vi "User Calibration New_without calibration.vi"(0 "CalStatusTab":T4(tab), 1 "SetDac In Process":bool, 5 "Processed Variables":T3 {"Chamber Temperature" format="%.2f"; "Ambient Temperature" format="%.2f"; "Bath Temperature" format="%.2f"; "Det. Temperature" format="%.2f"; "Detector Chl 4" format="%.2g"; "Detector Chl 3" format="%.2g"; "Ref CO2" format="%.2g"; "Detector Chl 2" format="%.2g"; "Film Temperature" format="%.2f"; "Humidity" format="%.2f"; "Detector Chl 1" format="%.2g"}, 9 "DACSet":u16[](array[numeric]) format="%03x", 11 "time_now":timestamp format="%<%H:%M:%S>T", 12 "Coefficients_In":T2[](array[typedef]) {"Elapsed Time" format="%<%H:%M:%S>t"; "zero_utc" format="%x"; "cal_utc" format="%x"; "Pump Flow Rate" format="%0d"; "Number of Zeroes" format="%0d"; "V2C" format="%0d"; "C2V" format="%0d"; "duration" format="%<%H:%M:%S>t"; "DAC" format="%03x"; "mI" format="%.3g"; "V_(RA,15mA)" format="%0.4f"; "V_(RA,5mA)" format="%0.4f"; "Chamber Temp" format="%.1f"; "Humidity" format="%.1f"}) -> (2 "Cal Fail":bool, 3 "Calibration Complete":bool, 4 "CalStatus Out":u16, 6 "DAC Currents":sgl[](array[numeric]) caption="Currents" format="%.4g", 8 "CalGasTank":u8=5 max=7, 10 "Pump Settings":T1, 14 "Coefficients_Out":T2[](array[typedef]) {"Elapsed Time" format="%<%H:%M:%S>t"; "zero_utc" format="%x"; "cal_utc" format="%x"; "Pump Flow Rate" format="%0d"; "Number of Zeroes" format="%0d"; "V2C" format="%0d"; "C2V" format="%0d"; "duration" format="%<%H:%M:%S>t"; "DAC" format="%03x"; "mI" format="%.3g"; "V_(RA,15mA)" format="%0.4f"; "V_(RA,5mA)" format="%0.4f"; "Chamber Temp" format="%.1f"; "Humidity" format="%.1f"}, 15 "SetDac":bool)   [LabVIEW 2015]
uses:
  <vilib>/Analysis/NI_AALBase.lvlib
  <vilib>/Analysis/baseanly.llb/Mean (DBL).vi
  Controls/Calibration Coefficients.ctl
  Controls/Processed Variables.ctl
  Controls/Pump Settings.ctl
panel:
  out "I_delta 2":dbl[](array[numeric]) format="%0.4f"
  out "Error":bool
  out "Index":u16
  out "null array":i16[][](array[numeric])
  out "stage 4 - offset adjust":i16[][](array[numeric])=[[0, 3, 500, 1, 1], [1, 3, 500, 1, 1], [2, 3, 500, 1, 1], [3, 3, 500, 1, 1], [4, 3, 500, 1, 1], [5, 3, 500, 1, 1], [6, 3, 500, 1, 1], [7, 3, 500, 0, 0], [8, 3, 500, 0, 0], [9, 3, 500, 0, 0], [10, 3, 500, 0, 0], [11, 3, 500, 0, 0], [12, 3, 500, 0, 0], [13, 3, 500, 0, 0], [14, 3, 500, 0, 0], [15, 3, 500, 0, 0], [16, 3, 500, 0, 0], [17, 3, 500, 0, 0], [18, 3, 500, 0, 0], [19, 3, 500, 0, 0], [20, 3, 500, 0, 0], [21, 3, 500, 0, 0], [22, 3, 500, 0, 0], [23, 3, 500, 0, 0], [24, 3, 500, 0, 0], [25, 3, 500, 0, 0], [26, 3, 500, 0, 0], [27, 3, 500, 0, 0], [28, 3, 500, 0, 0], [29, 3, 500, 0, 0], [30, 3, 500, 0, 0], [31, 3, 500, 0, 0], [32, 3, 500, 0, 0], [33, 3, 500, 0, 0], [34, 3, 500, 0, 0], [35, 3, 500, 0, 0], [36, 3, 500, 0, 0], [37, 3, 500, 0, 0], [38, 3, 500, 0, 0], [39, 3, 500, 0, 0], [40, 3, 500, 0, 0], [41, 3, 500, 0, 0], [42, 3, 500, 0, 0], [43, 3, 500, 0, 0], [44, 3, 500, 0, 0], [45, 3, 500, 0, 0], [46, 3, 500, 0, 0], [47, 3, 500, 0, 0], [48, 3, 500, 0, 0], [49, 3, 500, 0, 0], [50, 3, 500, 0, 0], [51, 3, 500, 0, 0], [52, 3, 500, 0, 0], [53, 3, 500, 0, 0], [54, 3, 500, 0, 0], [55, 3, 500, 0, 0], [56, 3, 500, 0, 0], [57, 3, 500, 0, 0], [58, 3, 500, 0, 0], [59, 3, 500, 0, 0], [60, 3, 500, 0, 0], [61, 3, 500, 0, 0], [62, 3, 500, 0, 0], [63, 3, 500, 0, 0], [64, 3, 500, 0, 0], [65, 3, 500, 0, 0], [66, 3, 500, 0, 0], [67, 3, 500, 0, 0], [68, 3, 500, 0, 0], [69, 3, 500, 0, 0], [70, 3, 500, 0, 0], [71, 3, 500, 0, 0], [72, 3, 500, 0, 0], [73, 3, 500, 0, 0], [74, 3, 500, 0, 0], [75, 3, 500, 0, 0], [76, 3, 500, 0, 0], [77, 3, 500, 0, 0], [78, 3, 500, 0, 0], [79, 3, 500, 0, 0], [80, 3, 500, 0, 0], [81, 3, 500, 0, 0], [82, 3, 500, 0, 0], [83, 3, 500, 0, 0], [84, 3, 500, 0, 0], [85, 3, 500, 0, 0], [86, 3, 500, 0, 0], [87, 3, 500, 0, 0], [88, 3, 500, 0, 0], [89, 3, 500, 0, 0], [90, 3, 500, 0, 0], [91, 3, 500, 0, 0], [92, 3, 50, 1, 1]]
  out "stage 3 - span":i16[][](array[numeric])=[[0, 3, 500, 0, 1], [1, 3, 500, 0, 1], [2, 3, 500, 0, 1], [3, 3, 500, 0, 1], [4, 3, 500, 0, 1], [5, 3, 500, 0, 1], [6, 3, 50, 0, 1]]
  out "stage 2 - zeroing":i16[][](array[numeric])=[[0, 2, 500, 1, 0], [1, 2, 500, 1, 0], [2, 2, 500, 1, 0], [3, 2, 500, 1, 0], [4, 2, 500, 1, 0], [5, 2, 500, 1, 0], [6, 2, 50, 1, 0]]
  out "stage1 - humidity check":i16[][](array[numeric])=[[0, 1, 500, 1, 0], [1, 1, 50, 1, 0], [2, 1, 50, 1, 0], [3, 1, 50, 1, 0], [4, 1, 50, 1, 0], [5, 1, 50, 1, 0], [6, 1, 100, 0, 1], [7, 1, 150, 0, 1], [8, 1, 200, 0, 1], [9, 1, 250, 1, 0], [10, 1, 300, 1, 1], [0, 1, 350, 0, 0]]
  out "Tcal_Film":dbl format="%.2f"
  out "I_delta":dbl[](array[numeric]) format="%0.4f"
  out "Actual":u16
  in  "Lo Flow":u16=50
  out "Tcal_Det":dbl[](array[numeric]) format="%.2f"
  out "Raw_Humidity":dbl format="%.2f"
  out "Raw Chamber":dbl format="%.2f"
  in  "Quit":bool
  in  "CalFile":path
  in  "Calfiles":string[](array[string])
  out "Reference":dbl format="%.3g"
  out "Tcal_Humidity":dbl format="%.2f"
  in  "Hi Flow Setting":u16=100
  out "Progress Out":u8(slide) scale=0.0..255.0
  in  "Progress":u16(slide) scale=0.0..666.0
  out "Cal Gas":dbl=nan format="%.3g"
  in  "Skip Cal":bool
  in  "OK  7":bool
  in  "Calgas":dbl caption="Calibration Gas Concentration" format="%.2g"
  out "start time":timestamp format="%<%H:%M:%S>T"
  in  "Gas Tank":u8=5
  out "Calibration Message":enum16{"Calibration Is Required - "}(ring)
  in  "Calibration Code":T5(ring)
  out "Stable":bool
  in  "Low Humidity Threshold (%)":u16=60
  in  "Hi Humidity Threshold (%)":u16=90
  in  "Humidity Status":T6(ring)
  out "Stablizing":dbl[][](graph)
  out "Status":bool[](array[boolean])
  out "V2C":u8[](array[numeric])
  out "D'":dbl[](array[numeric]) format="%0.4f"
  out "C'":dbl[](array[numeric]) format="%0.4f"
  out "B'":dbl[](array[numeric]) format="%0.4f"
  out "A'":dbl[](array[numeric]) format="%0.4f"
  out "D":dbl[](array[numeric]) format="%0.4f"
  out "C":dbl[](array[numeric]) format="%0.4f"
  out "B":dbl[](array[numeric]) format="%0.4f"
  out "A":dbl[](array[numeric]) format="%0.4f"
  out "C2V":u8[](array[numeric])
  out "CHANNEL":string[](array[string])
  out "C0FC2V":dbl[](array[numeric]) format="%0.4f"
  out "C6FC2V":dbl[](array[numeric]) format="%0.4f"
  out "TYPE":string
  out "DATE":string
  out "CalFile Selected":path
  out "V_0d(target)":dbl[](array[numeric]) format="%0.4f"
  out "V_6d(target)":dbl[](array[numeric]) format="%0.4f"
  out "V_span(target)":dbl[](array[numeric]) format="%0.4f"
  out "BlueLED 2":bool[](array[boolean]) caption="BlueLED"
  out "DAC scale":dbl[](array[numeric]) format="%.3g"
  out "Zero":dbl[][](graph)
  out "Zero Status":T7(ring)
  out "V_RA(5mA)":dbl[](array[numeric]) format="%0.4f"
  out "V_RA(15mA)":dbl[](array[numeric]) format="%0.4f"
  out "mI":dbl[](array[numeric]) format="%.3g"
  out "delta 2":dbl=nan caption="delta" format="%.3g"
  out "CHANNEL 2":string[](array[string]) caption="CHANNEL"
  out "BlueLED":bool[](array[boolean])
  out "Zero 3":dbl[][](graph)
  out "CHANNEL 3":string[](array[string]) caption="CHANNEL"
  out "BlueLED 3":bool[](array[boolean]) caption="BlueLED"
  out "I'mBlue 2":bool[](array[boolean]) caption="BlueLED"
  out "V_RA(5mA) 2":dbl[](array[numeric]) format="%0.4f"
  out "V_RA(15mA) 2":dbl[](array[numeric]) format="%0.4f"
  out "mI 2":dbl[](array[numeric]) format="%.3g"
  out "DAC scale 2":dbl[](array[numeric]) format="%.3g"
  out "delta 3":dbl=nan caption="delta" format="%.3g"
  out "Zero Status 2":T8(ring)
  in  "OK 9":bool
  out "I_span":dbl[](array[numeric]) format="%0.4f"
  out "Step":i16[](array[numeric])
  out "DAC":u16[](array[numeric]) format="%03x"
  out "V_Span Delta":dbl[](array[numeric]) format="%0.4f"
  out "Span Good":bool[](array[boolean])
  out "I'mBlue":bool[](array[boolean]) caption="BlueLED"
  out "Span Point Calibration":dbl[][](graph)
  out "delta":dbl=nan format="%.3g"
  out "Zero Offset":dbl[][](graph)
  in  "OK 10":bool
  out "Calibration Complete -":timestamp format="%<%H:%M:%S\n%m/%d/%y>T"
  out "duration":i16 caption="mins" format="%<%H:%M:%S>t"
  out "V_0d(ImA)":dbl[](array[numeric]) format="%0.4f"
  out "V_6d(ImA)":dbl[](array[numeric]) format="%0.4f"
  out "V_0(adjust)":dbl[](array[numeric]) format="%0.4f"
  out "V_span(adjust)":dbl[](array[numeric]) format="%0.4f"
  out "Gain(adjust)":dbl[](array[numeric]) format="%0.4f"
  out "V_span(ImA)":dbl[](array[numeric]) format="%0.4f"
  out "Tcal_PCB":dbl=nan format="%.2f"
  out "Tcal_Chamber":dbl format="%.2f"
  out "elapsed time":i16 format="%<%H:%M:%S>t"
  out "Count":u8
  # "Channel 1"
  # "Channel 2"
  # "Channel 3"
  # "Channel 4"
  # "Initializing"
  # "1. Please Place Freespira On Base-Station\n \n2. Attach Cannula and Breathe Normally \n \n3. Enter Calibration Gas Concentration \n \n4. Press OK To Begin Calibration Process"
  # "Please Enter Calibration Code"
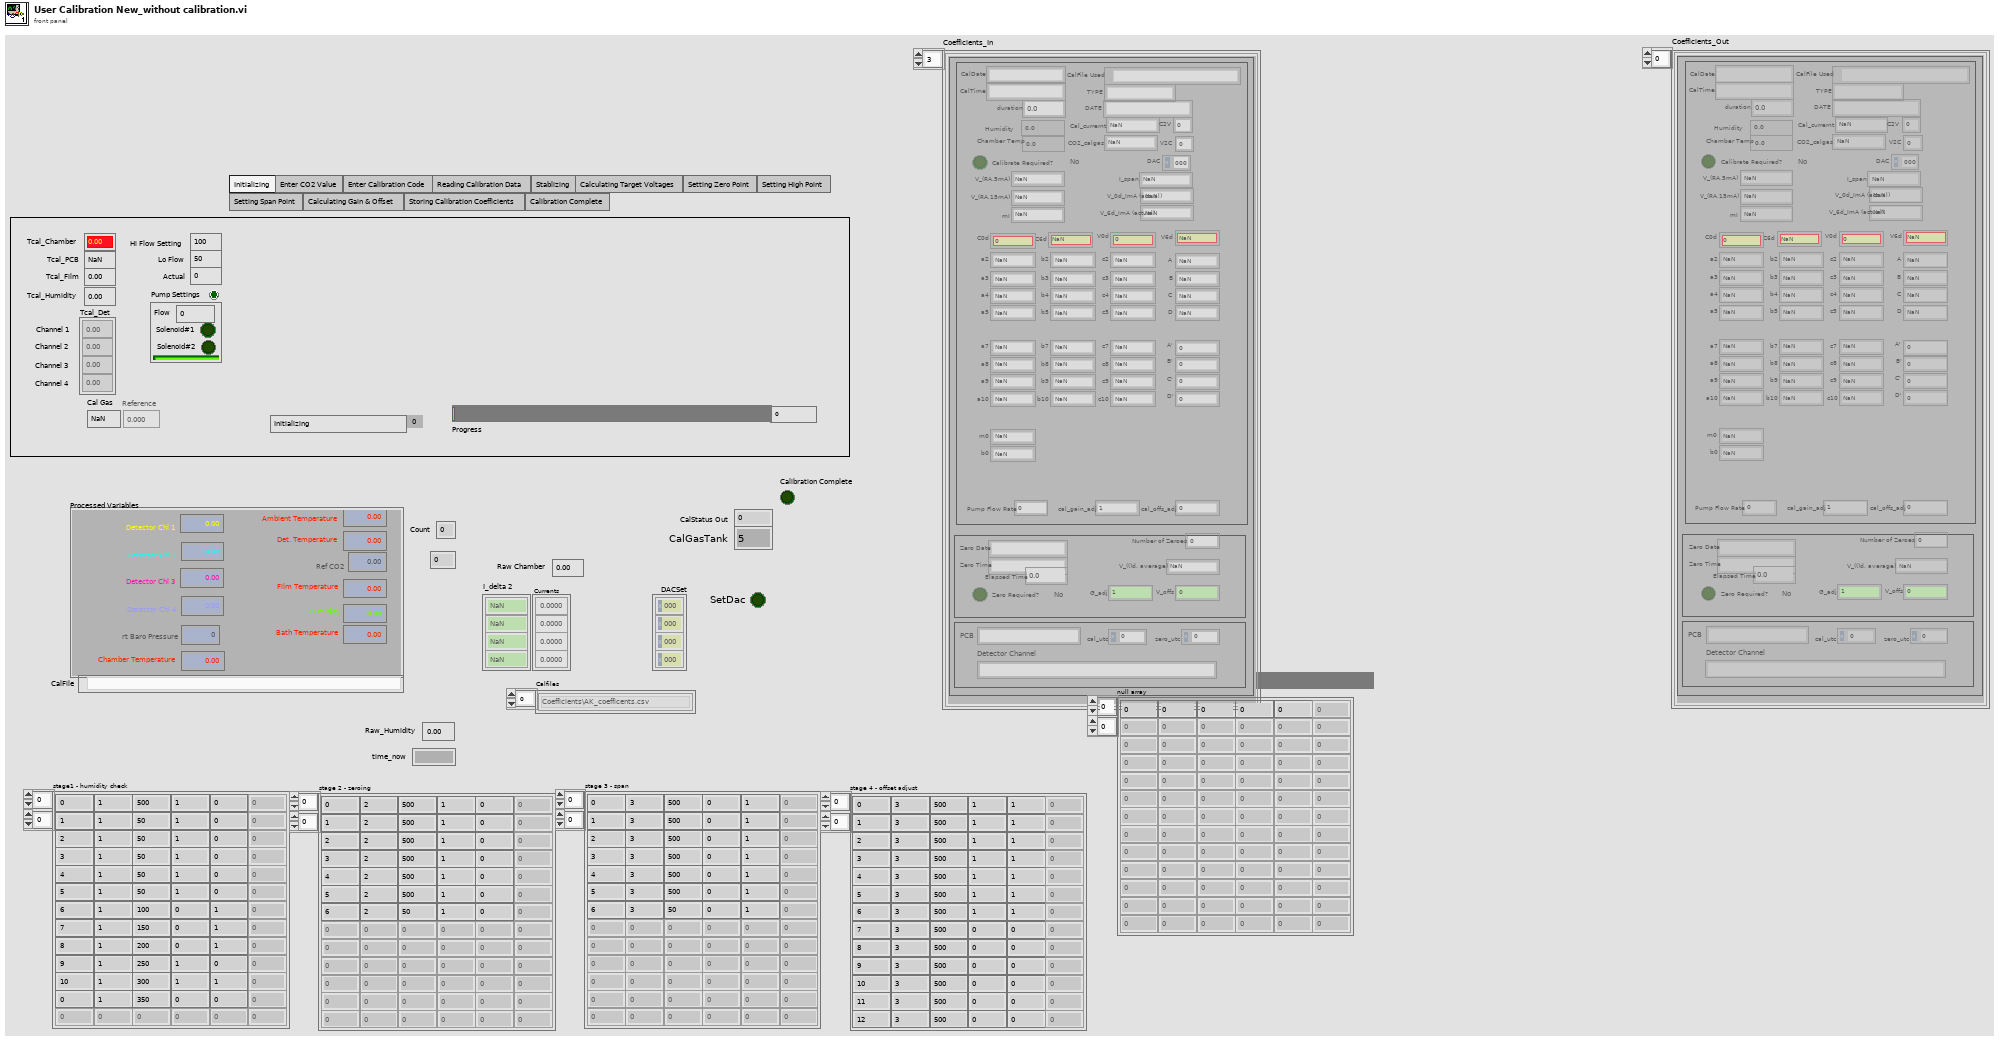
[diagram p1: front panel]
types:
  T1 = typedef "Pump Settings.ctl" = cluster{"Flow":u16, "Solenoid#1":bool, "Solenoid#2":bool, "ignore":bool}
  T2 = typedef "Calibration Coefficients.ctl" = cluster{"CalFile Used":path, "TYPE":string, "DATE":string, "Humidity":sgl, "Chamber Temp":dbl, "CO2_calgas":dbl, "V_(RA,5mA)":dbl, "V_(RA,15mA)":dbl, "mI":dbl, "V_0d_ImA (actual)":dbl, "V_6d_ImA (actual)":dbl, "I_span":dbl, "DAC":u16, "A":dbl, "B":dbl, "C":dbl, "D":dbl, "V6d":dbl, "A'":dbl, "B'":dbl, "C'":dbl, "D'":dbl, "V0d":dbl, "CalDate":string, "CalTime":string, "duration":dbl, "Detector Channel":string, "a2":dbl, "a3":dbl, "a4":dbl, "a5":dbl, "b2":dbl, "c2":dbl, "b3":dbl, "c3":dbl, "b4":dbl, "c4":dbl, "b5":dbl, "c5":dbl, "a7":dbl, "a8":dbl, "a9":dbl, "a10":dbl, "b7":dbl, "b8":dbl, "b9":dbl, "b10":dbl, "c7":dbl, "c8":dbl, "c9":dbl, "c10":dbl, "cal_offs_adj":dbl, "cal_gain_adj":dbl, "C6d":dbl, "C0d":dbl, "Cal_currernt":dbl, "C2V":u16, "V2C":u16, "Zero Date":string, "Zero Time":string, "Number of Zeroes":u16, "V_(()d, average)":dbl, "V_offs ":dbl, "G_adj":dbl, "Pump Flow Rate":u16, "Zero Required? ":bool, "Calibrate Required?":bool, "cal_utc":dbl, "zero_utc":dbl, "Elapsed Time":dbl, "PCB":string, "m0":dbl, "b0":dbl}
  T3 = typedef "Processed Variables.ctl" = cluster{"Detector Chl 1":sgl, "Humidity":dbl, "Film Temperature":dbl, "Detector Chl 2":sgl, "Ref CO2":sgl, "Detector Chl 3":sgl, "Detector Chl 4":sgl, "Det. Temperature":dbl, "Bath Temperature":dbl, "Ambient Temperature":dbl, "rt Baro Pressure":u16, "Chamber Temperature":dbl}
  T4 = enum32{"Initializing", "Enter CO2 Value", "Enter Calibration Code", "Reading Calibration Data", "Stablizing", "Calculating Target Voltages", "Setting Zero Point", "Setting High Point", "Setting Span Point", "Calculating Gain & Offset", "Storing Calibration Coefficients", "Calibration Complete"}
  T5 = enum8{"", "<User Defined>", "11111 - default", "22222 - MM_1_NS", "33333 - MM_2_S"}
  T6 = enum16{"Waiting For Film to Stabilize", "Film Stable", "Exiting", "Initializing"}
  T7 = enum16{"Setting Zero at 5 mA", "Setting Zero at 15 mA", "Calculating slopes"}
  T8 = enum16{"Setting High at 5 mA", "Setting High at 15 mA", "Calculating slopes"}
  T9 = enum32{"Invalid", "Standard", "Closed", "Hidden", "Minimized", "Maximized"}
  T10 = enum16{"Waiting For Film to Stabilize", "Film Stable - Press OK to Continue", "Exiting"}
  T11 = enum16{"Waiting For Film to Stabilize", "Film Stable - Press OK to Continue", "Exiting", "Initializing"}
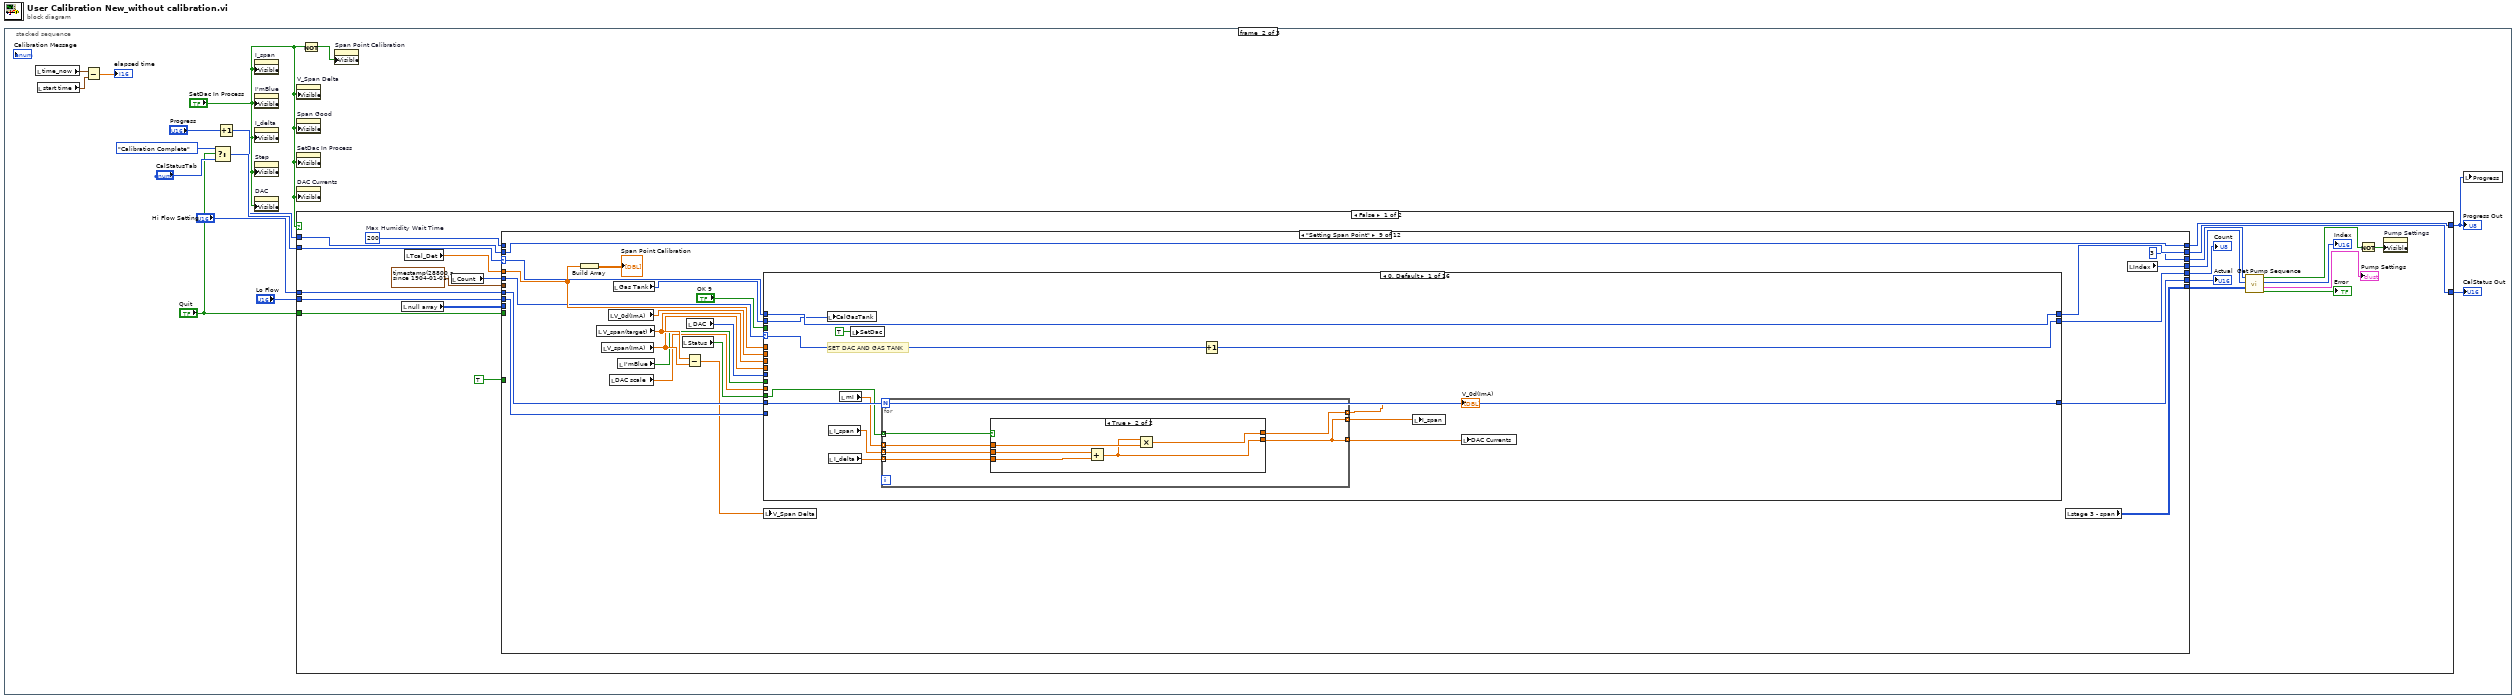
[diagram p0: block diagram]
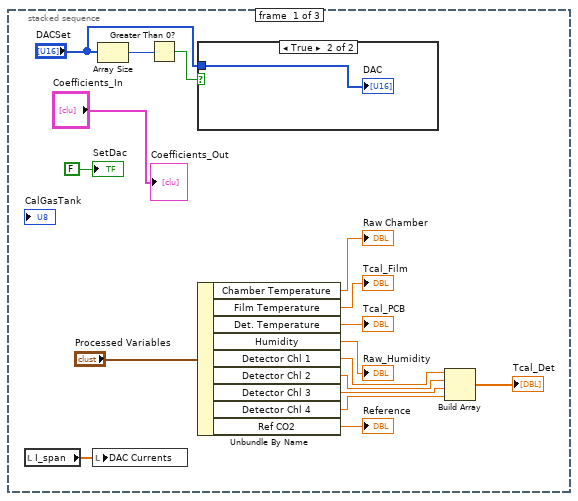
[diagram p2: hidden frame]
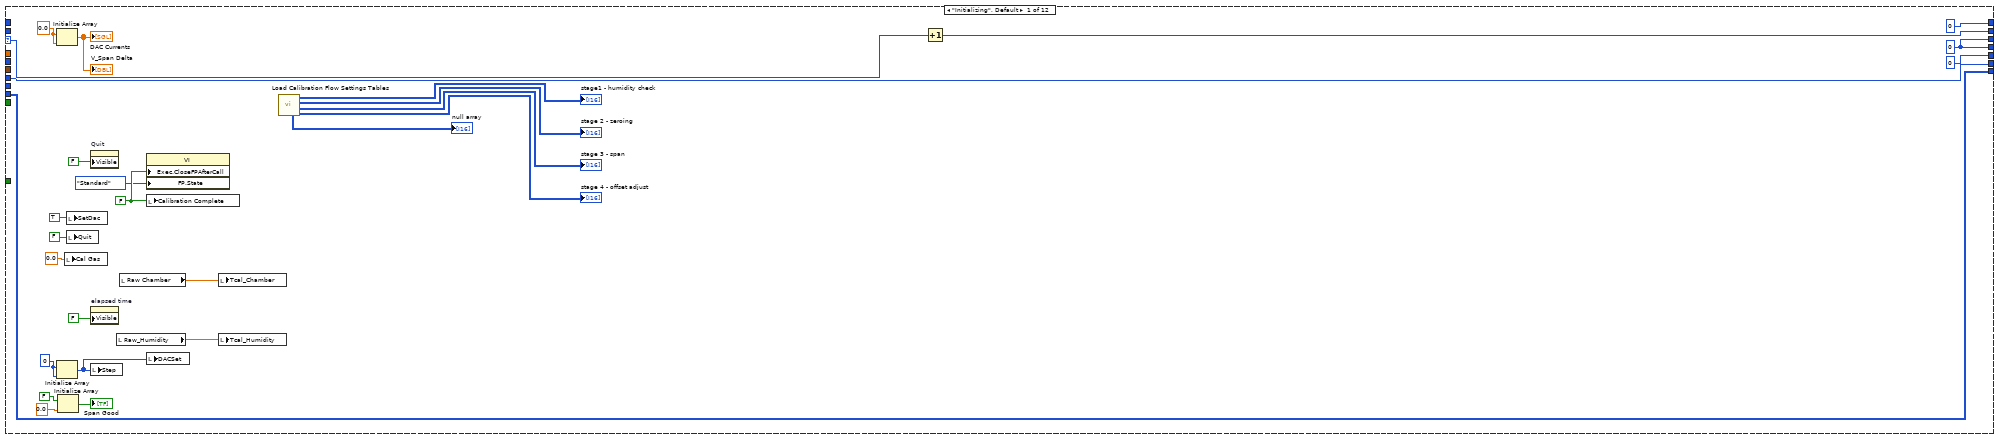
[diagram p4: hidden frame]
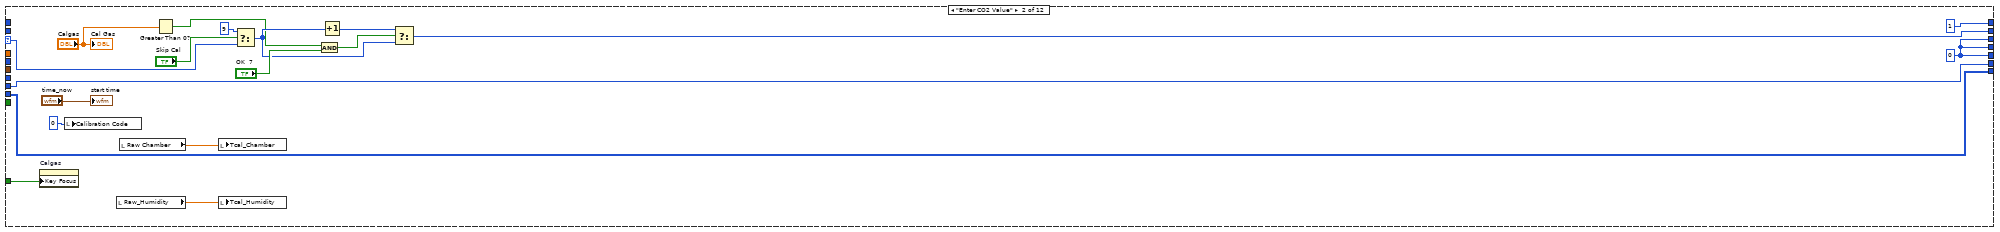
[diagram p5: hidden frame]
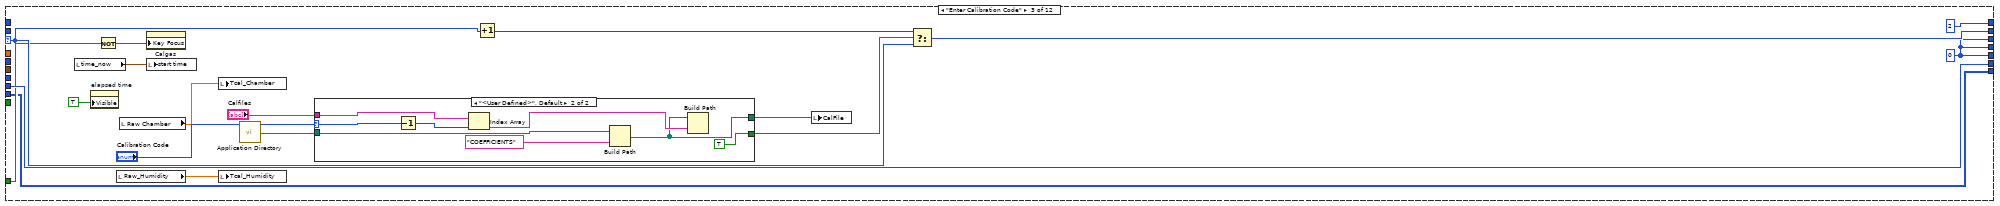
[diagram p6: hidden frame]
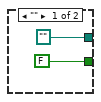
[diagram p7: hidden frame]
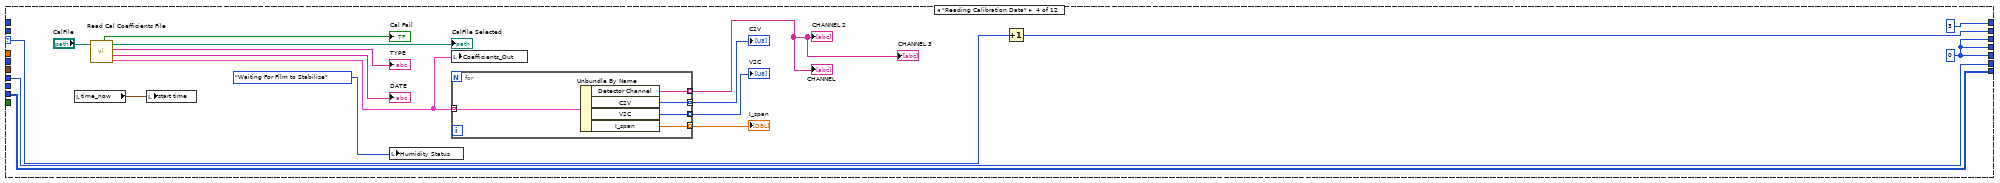
[diagram p8: hidden frame]
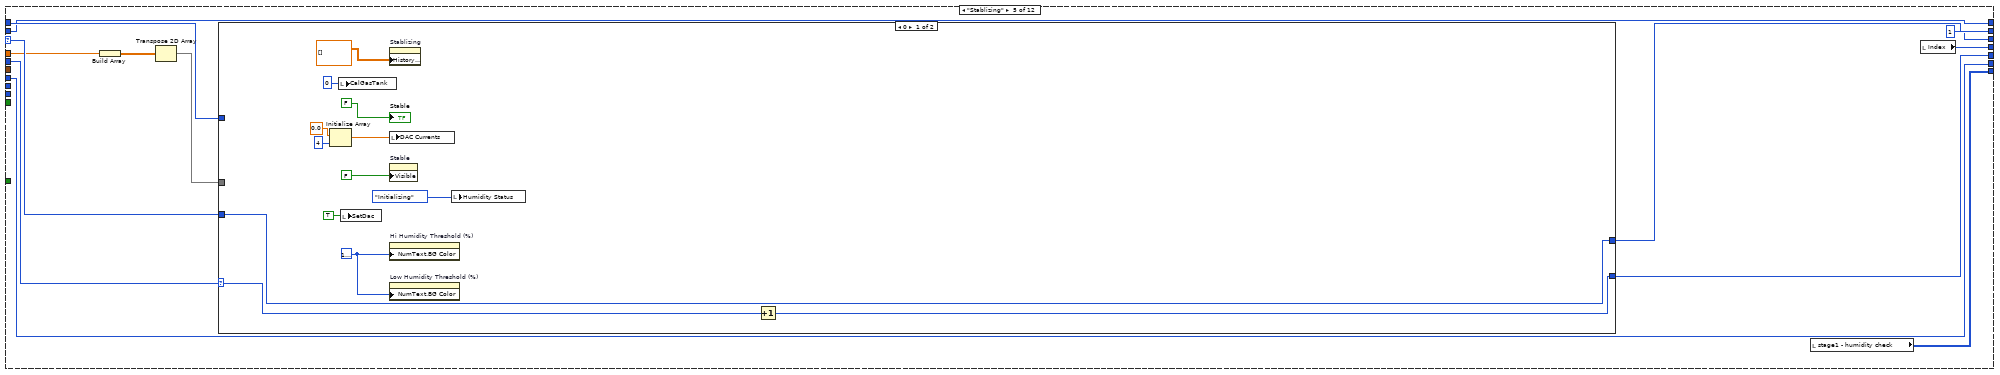
[diagram p9: hidden frame]
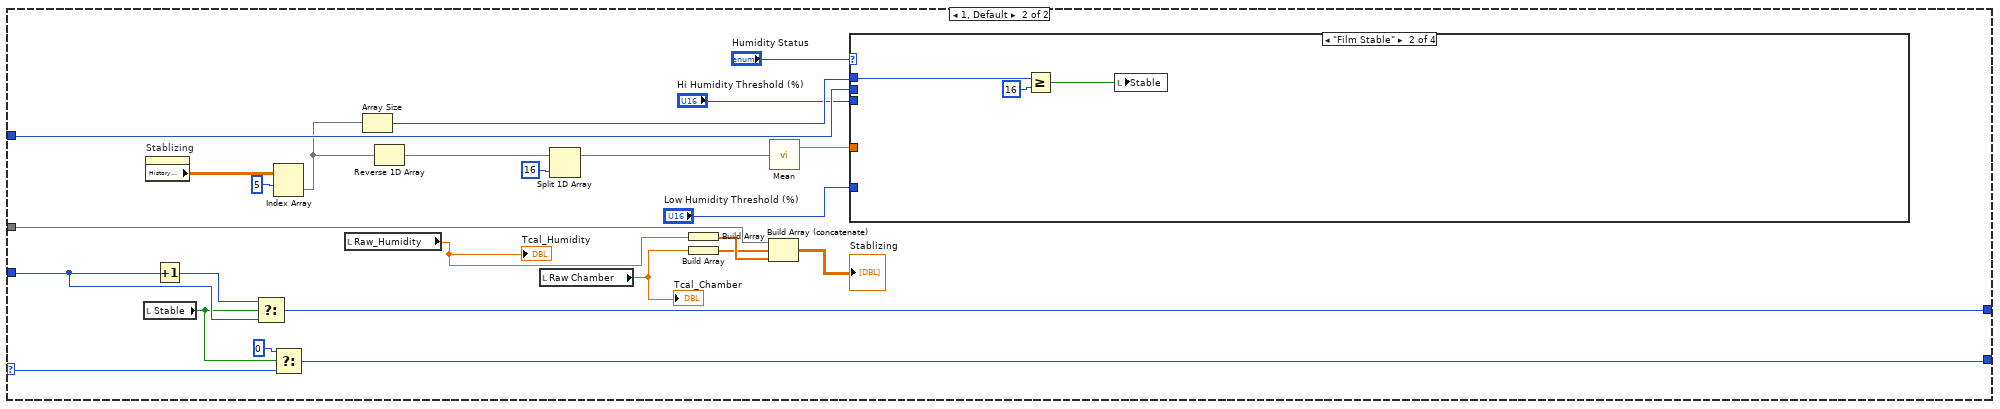
[diagram p10: hidden frame]
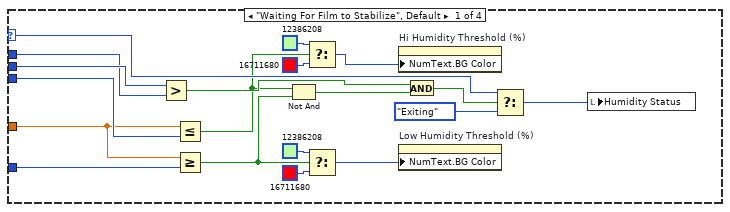
[diagram p11: hidden frame]
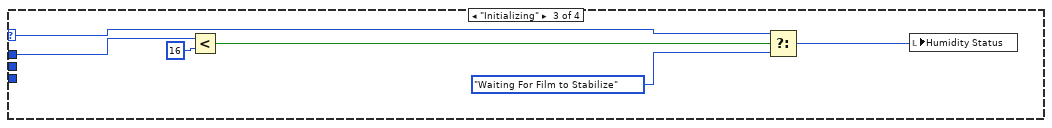
[diagram p12: hidden frame]
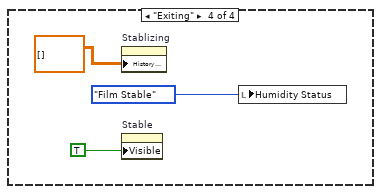
[diagram p13: hidden frame]
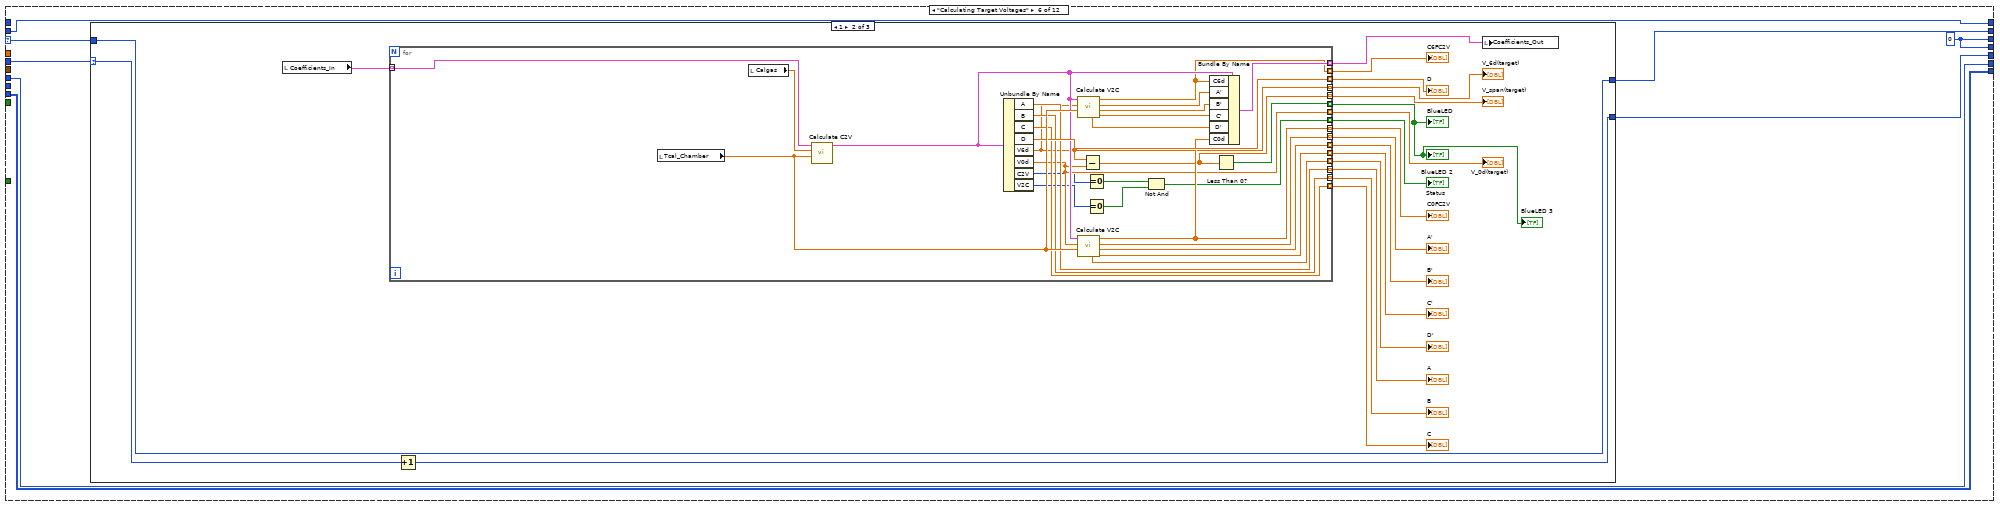
[diagram p14: hidden frame]
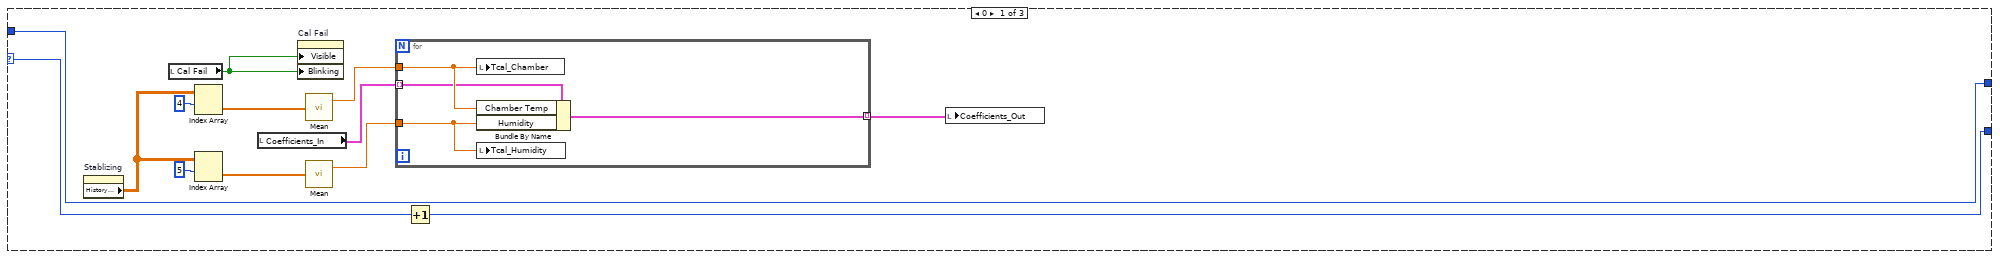
[diagram p15: hidden frame]
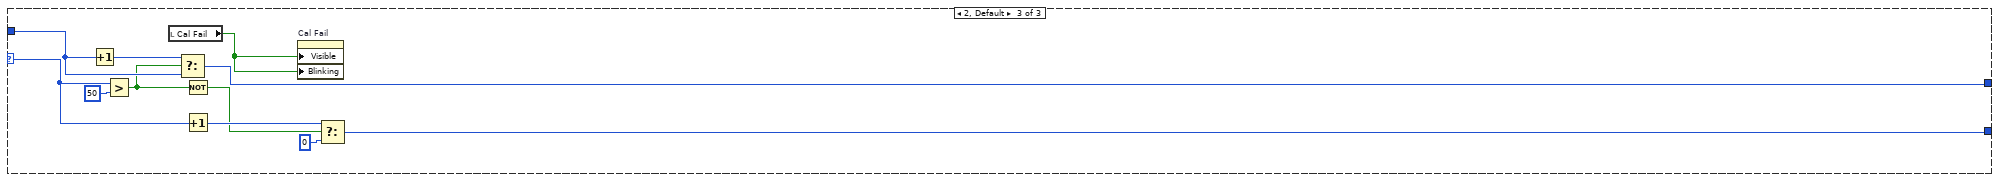
[diagram p16: hidden frame]
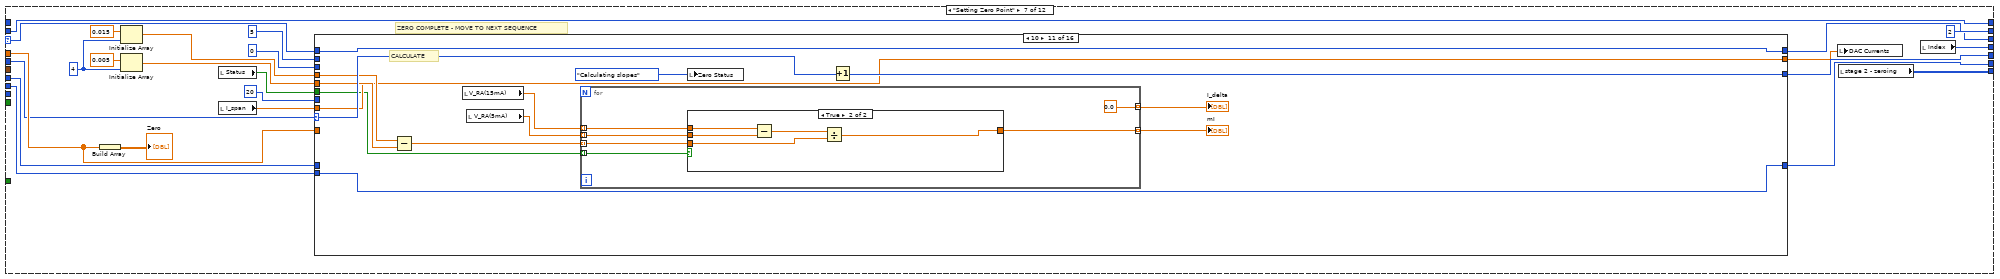
[diagram p17: hidden frame]
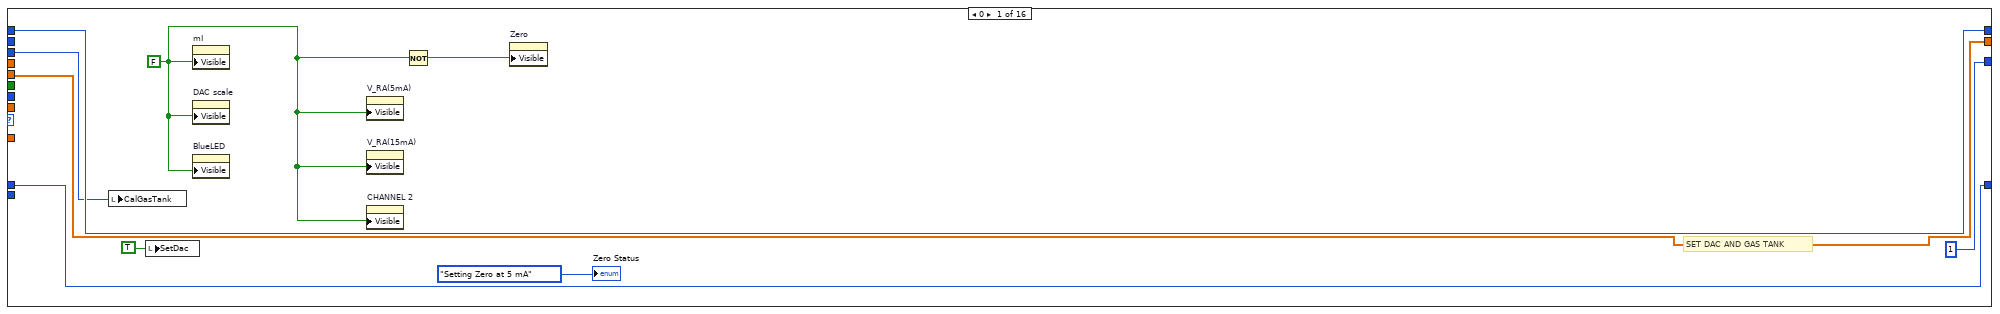
[diagram p18: hidden frame]
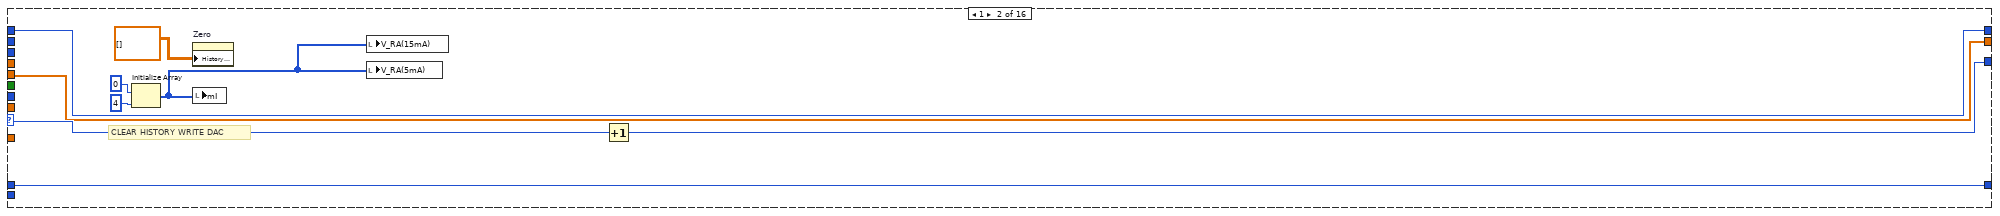
[diagram p19: hidden frame]
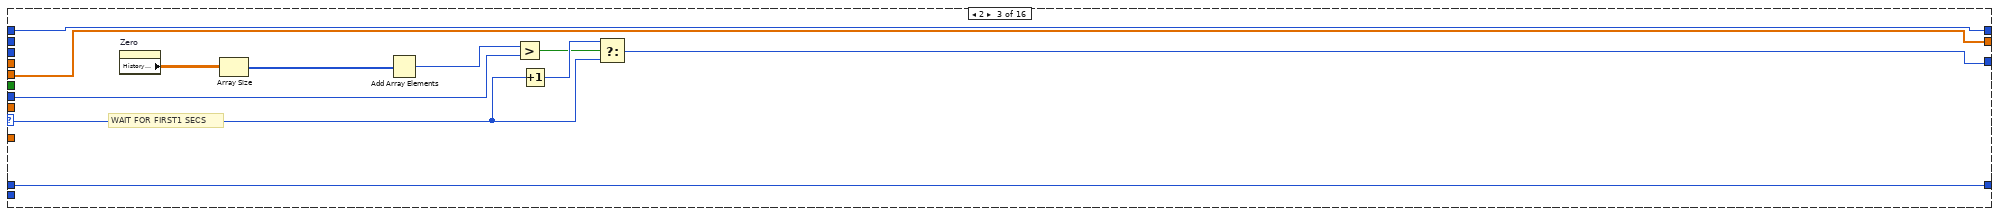
[diagram p20: hidden frame]
diagram:
  n1 = stacked-sequence {
    frame #0 {
      n2 = local read "I_span"() -> (w4:dbl[])
      n3 = local write "DAC Currents"(w4) -> ()
      n4 = Array Size(array="DACSet") -> (size(s)=w6:i32)
      n5 = Greater Than 0?(x=w6) -> (x > 0?=w5:bool)
      n6 = case shown="True" w5 {
        tunnel: "DACSet" -> [_ w18]
        frame False {
        }
        frame True {
          "DAC" <- w18
        }
      }
      n7 = Unbundle By Name("Processed Variables") -> ("Chamber Temperature"=→"Raw Chamber":dbl, "Film Temperature"=→"Tcal_Film":dbl, "Det. Temperature"=→"Tcal_PCB":dbl, "Humidity"=→"Raw_Humidity":dbl, "Detector Chl 1"=w10:sgl, "Detector Chl 2"=w9:sgl, "Detector Chl 3"=w8:sgl, "Detector Chl 4"=w12:sgl, "Ref CO2"=→"Reference":sgl)
      n8 = Build Array(w10, w9, w8, w12) -> (→"Tcal_Det":sgl[])
      "SetDac" <- FALSE
      "Coefficients_Out" <- "Coefficients_In"
    }
    frame #1 {
      n9 = local read "time_now"() -> (w29:timestamp)
      n10 = local read "start time"() -> (w30:timestamp)
      n11 = Subtract(x=w29, y=w30) -> (x-y=→"elapsed time":dbl)
      n12 = Select(t=T4."Calibration Complete" ("CalStatusTab"), s="Quit", f="CalStatusTab") -> (s? t:f=w25:T4)
      n13 = Increment(x="Progress") -> (x+1=w24:u16)
      n14 = property on="I_span" class="Arr (strict)"("Visible"="SetDac In Process") -> ()  [unwired: 2 in, 2 out]
      n15 = property on="I'mBlue" class="Arr (strict)"("Visible"="SetDac In Process") -> ()  [unwired: 2 in, 2 out]
      n16 = property on="I_delta" class="Arr (strict)"("Visible"="SetDac In Process") -> ()  [unwired: 2 in, 2 out]
      n17 = property on="Step" class="Arr (strict)"("Visible"="SetDac In Process") -> ()  [unwired: 2 in, 2 out]
      n18 = property on="DAC" class="Arr (strict)"("Visible"="SetDac In Process") -> ()  [unwired: 2 in, 2 out]
      n19 = property on="V_Span Delta" class="Arr (strict)"("Visible"="SetDac In Process") -> ()  [unwired: 2 in, 2 out]
      n20 = property on="Span Good" class="Arr (strict)"("Visible"="SetDac In Process") -> ()  [unwired: 2 in, 2 out]
      n21 = property on="SetDac In Process" class="Bool (strict)"("Visible"="SetDac In Process") -> ()  [unwired: 2 in, 2 out]
      n22 = property on="DAC Currents" class="Arr (strict)"("Visible"="SetDac In Process") -> ()  [unwired: 2 in, 2 out]
      n23 = case shown="False" "SetDac In Process" {
        tunnel: [w56 w1350] -> w33
        tunnel: [w55 w1349] -> w31
        tunnel: "Quit" -> [w51 _]
        tunnel: w25 -> [w50 w1349]
        tunnel: w24 -> [w49 w1350]
        tunnel: "Lo Flow" -> [w45 _]
        tunnel: "Hi Flow Setting" -> [w44 _]
        frame False {
          w54 = 200  # Max Humidity Wait Time
          n24 = local read "null array"() -> (w42:i16[][])
          n25 = local read "Tcal_Det"() -> (w47:dbl[])
          n26 = local read "Count"() -> (w53:u8)
          n27 = case shown="\"Setting Span Point\"" w50 {
            selector: w50 -> [w84 w93 w118 w149 w165 w244 w344 w593 w853 w1159 w1259 w1344]
            tunnel: [w80 w103 w121 w147 w164 w243 w343 w592 w852 w1158 w1258 w1344] -> w55
            tunnel: w49 -> [_ _ _ _ w163 w239 w342 w591 w851 w1160 w1257 w1343]
            tunnel: [0 1 2 3 w163 w239 w342 w591 w851 w1160 w1256 w1342] -> w56
            tunnel: w51 -> [_ _ _ _ _ _ _ _ _ _ _ _]
            tunnel: w45 -> [_ w96 w113 _ _ _ w337 w587 w848 w1153 w1255 w1340]
            tunnel: w44 -> [w77 _ _ w144 w159 w240 w336 w586 w847 w1154 _ _]
            tunnel: w54 -> [_ _ _ _ w166 _ _ _ _ _ _ _]
            tunnel: w53 -> [_ _ _ _ w158 w242 w324 w575 w835 w1147 w1254 w1341]
            tunnel: [u8 0 w85 w104 w133 w167 w241 w338 w588 w849 w1157 w1253 w1341] -> w48
            tunnel: [w77 w96 w113 w144 w159 w240 w335 w585 w846 w1156 w1252 w1340] -> w46
            tunnel: timestamp(28800 s since 1904-01-01) -> [_ _ _ _ _ _ _ _ _ _ w1251 _]
            tunnel: w47 -> [_ _ _ _ w162 _ w334 w584 w844 w1151 _ _]
            tunnel: TRUE ("Key Focus") -> [_ w87 w109 _ _ _ _ _ _ _ _ _]
            tunnel: [w58 w86 w105 w134 w157 w238 w323 w574 w834 w1148 w1250 w1338] -> w38
            tunnel: w42 -> [w58 w86 w105 w134 _ w238 _ _ _ _ w1250 w1338]
            tunnel: [w57 w85 w104 w133 1 w237 2 ("Count") 2 ("Count") 3 ("Count") 4 ("Count") w1249 w1337] -> w41
            tunnel: [w57 w85 w104 w133 w156 w237 w321 w572 w833 w1146 w1249 w1337] -> w40
            frame "Initializing", Default {
              w57 = 0
              w70 = 0.0
              w72 = 0
              w82 = FALSE ("Calibration Complete")
              n28 = Initialize Array(w70, w70) -> (→"V_Span Delta" →"DAC Currents":dbl[])
              n29 = Initialize Array(w72, w72) -> (w65:i32[])
              n30 = Initialize Array(FALSE, 0.0) -> (→"Span Good":bool[])
              n31 = local write "Cal Gas"(0.0) -> ()
              n32 = local write "SetDac"(TRUE ("SetDac")) -> ()
              n33 = local write "Quit"(FALSE ("Cal Fail")) -> ()
              n34 = property on="Quit" class="Bool (strict)"("Visible"=FALSE ("Blinking")) -> ()  [unwired: 2 in, 2 out]
              n35 = property on="elapsed time" class="DigNum (strict)"("Visible"=FALSE) -> ()  [unwired: 2 in, 2 out]
              n36 = local write "Step"(w65) -> ()
              n37 = local read "Raw_Humidity"() -> (w75:dbl)
              n38 = local read "Raw Chamber"() -> (w74:dbl)
              n39 = property class="VI"("Exec.CloseFPAfterCall"=w82, "FP.State"=T9."Standard" ("Front Panel Window:State")) -> ()  [unwired: 2 in, 2 out]
              n40 = local write "Calibration Complete"(w82) -> ()
              n41 = local write "DACSet"(w65) -> ()
              n42 = local write "Tcal_Chamber"(w74) -> ()
              n43 = local write "Tcal_Humidity"(w75) -> ()
              n44 = call "Load Calibration Flow Settings Tables.vi"() -> ("stage 4 - span"=→"stage 4 - offset adjust":i16[][], "stage 3 - high"=→"stage 3 - span":i16[][], "stage 2 - zeroing"=→"stage 2 - zeroing":i16[][], "stage1 - humidity check"=→"stage1 - humidity check":i16[][], "stage 5 - offset adjust"=→"null array":i16[][])  [unwired: 6 in, 1 out]
              n45 = Increment(x=w84) -> (x+1=w80:T4)
            }
            frame "Enter CO2 Value" {
              w85 = u8 0
              n46 = property on="Calgas" class="DigNum (strict)"("Key Focus"=w87) -> ()  [unwired: 2 in, 2 out]
              n47 = local write "Calibration Code"(0) -> ()
              n48 = local read "Raw_Humidity"() -> (w90:dbl)
              n49 = local read "Raw Chamber"() -> (w89:dbl)
              n50 = Greater Than 0?(x="Calgas") -> (x > 0?=w88:bool)
              n51 = local write "Tcal_Chamber"(w89) -> ()
              n52 = local write "Tcal_Humidity"(w90) -> ()
              n53 = Select(t=u16 9 ("CalStatus Out"), s="Skip Cal", f=w93) -> (s? t:f=w94:u32)
              n54 = And(x=w88, y="OK  7") -> (x .and. y?=w97:bool)
              n55 = Increment(x=w94) -> (x+1=w102:u32)
              n56 = Select(t=w102, s=w97, f=w94) -> (s? t:f=w103:u32)
              "start time" <- "time_now"
              "Cal Gas" <- "Calgas"
            }
            frame "Enter Calibration Code" {
              w104 = u8 0
              n57 = local read "time_now"() -> (w110:timestamp)
              n58 = property on="elapsed time" class="DigNum (strict)"("Visible"=TRUE) -> ()  [unwired: 2 in, 2 out]
              n59 = Not(x=w109) -> (.not. x?=w108:bool)
              n60 = local read "Raw_Humidity"() -> (w112:dbl)
              n61 = local read "Raw Chamber"() -> (w111:dbl)
              n62 = property on="Calgas" class="DigNum (strict)"("Key Focus"=w108) -> ()  [unwired: 2 in, 2 out]
              n63 = local write "start time"(w110) -> ()
              n64 = local write "Tcal_Chamber"(w111) -> ()
              n65 = local write "Tcal_Humidity"(w112) -> ()
              n66 = call <vilib>:"Application Directory.vi"() -> ("Application Directory"=w107:path)
              n67 = case shown="\"<User Defined>\", Default" "Calibration Code" {
                selector: "Calibration Code" -> [_ w129]
                tunnel: [FALSE TRUE] -> w117
                tunnel: "Calfiles" -> [_ w130]
                tunnel: w107 -> [_ w126]
                tunnel: [path "" w124] -> w106
                frame "" {
                }
                frame "<User Defined>", Default {
                  n68 = Decrement(x=w129) -> (x-1=w128:T5)
                  n69 = Index Array(array=w130, index=w128) -> (element=w131:string)
                  n70 = Build Path(base path=w126, name or relative path="COEFFICIENTS") -> (appended path=w124:path)
                  n71 = Build Path(base path=w124, name or relative path=w131) -> ()  [unwired: 1 out]
                }
              }
              n72 = Increment(x=w118) -> (x+1=w120:T4)
              n73 = local write "CalFile"(w106) -> ()
              n74 = Select(t=w120, s=w117, f=w118) -> (s? t:f=w121:T4)
            }
            frame "Reading Calibration Data" {
              w133 = u8 0
              n75 = local read "time_now"() -> (w145:timestamp)
              n76 = call "Read Cal Coefficients File.vi"(11:"CalFile") -> ("Original Coefficients"=w140:T2[], "DATE"=→"DATE":string, "TYPE"=→"TYPE":string, "CalFile Selected"=→"CalFile Selected":path, "Error"=→"Cal Fail":bool)  [unwired: 5 in, 1 out]
              n77 = local write "start time"(w145) -> ()
              n78 = local write "Humidity Status"(enum16{"Waiting For Film to Stabilize"}."Waiting For Film to Stabilize" ("Enum")) -> ()
              n79 = local write "Coefficients_Out"(w140) -> ()
              n80 = for {
                tunnel: w140 -> [w154] mode=indexing
                tunnel: [w153] -> w137 mode=indexing
                tunnel: [w152] -> w136 mode=indexing
                tunnel: [w151] -> w135 mode=indexing
                tunnel: [w150] -> w132 mode=indexing
                n81 = Unbundle By Name(w154) -> ("Detector Channel"=w150:string, "C2V"=w151:u16, "V2C"=w152:u16, "I_span"=w153:dbl)
              }
              "I_span" <- w137
              "V2C" <- w136
              "C2V" <- w135
              "CHANNEL" <- w132
              "CHANNEL 2" <- w132
              "CHANNEL 3" <- w132
              n82 = Increment(x=w149) -> (x+1=w147:T4)
            }
            frame "Stablizing" {
              n83 = Build Array(w162) -> (w161:dbl[][])
              n84 = Transpose 2D Array(2D array=w161) -> (transposed array=w160:dbl[][])
              n85 = case shown="0" w158 {
                selector: w158 -> [w180 w200]
                tunnel: [w179 w201] -> w167
                tunnel: w166 -> [_ w195]
                tunnel: w165 -> [w178 w199]
                tunnel: [w178 w198] -> w164
                tunnel: w160 -> [_ w182]
                frame 0 {
                  w172 = u32 16777216
                  n86 = Initialize Array(0.0, 4 ("dimension size")) -> (w170:dbl[])
                  n87 = local write "CalGasTank"(u8 0 ("CalGasTank")) -> ()
                  n88 = local write "SetDac"(TRUE ("InCal")) -> ()
                  n89 = property on="Stablizing" class="WFChart (strict)"("History Data"=dbl[][] []) -> ()  [unwired: 2 in, 2 out]
                  n90 = local write "DAC Currents"(w170) -> ()
                  n91 = property on="Stable" class="Bool (strict)"("Visible"=FALSE) -> ()  [unwired: 2 in, 2 out]
                  n92 = property on="Hi Humidity Threshold (%)" class="DigNum (strict)"("NumText.BG Color"=w172) -> ()  [unwired: 2 in, 2 out]
                  n93 = property on="Low Humidity Threshold (%)" class="DigNum (strict)"("NumText.BG Color"=w172) -> ()  [unwired: 2 in, 2 out]
                  n94 = local write "Humidity Status"(T6."Initializing" ("Humidity Status")) -> ()
                  n95 = Increment(x=w180) -> (x+1=w179:u8)
                  "Stable" <- FALSE ("Done")
                }
                frame 1, Default {
                  n96 = local read "Stable"() -> (w181:bool)
                  n97 = property on="Stablizing" class="WFChart (strict)"() -> ("History Data"=w203:dbl[][])  [unwired: 2 in, 2 out]
                  n98 = Increment(x=w199) -> (x+1=w202:T4)
                  n99 = Select(t=w202, s=w181, f=w199) -> (s? t:f=w198:T4)
                  n100 = Index Array(array=w203, index (row)=5) -> (element=w190:dbl[])  [unwired: 1 in]
                  n101 = Select(t=u8 0, s=w181, f=w200) -> (s? t:f=w201:u8)
                  n102 = local read "Raw_Humidity"() -> (w184:dbl)
                  "Tcal_Humidity" <- w184
                  n103 = Array Size(array=w190) -> (size(s)=w197:i32)
                  n104 = Reverse 1D Array(array=w190) -> (reversed array=w191:dbl[])
                  n105 = local read "Raw Chamber"() -> (w183:dbl)
                  "Tcal_Chamber" <- w183
                  n106 = Split 1D Array(array=w191, index=16) -> (first subarray=w192:dbl[])  [unwired: 1 out]
                  n107 = Build Array(w184) -> (w187:dbl[])
                  n108 = Build Array(w183) -> (w185:dbl[])
                  n109 = Build Array (concatenate)(w182, w185, w187) -> (→"Stablizing":dbl[][])
                  n110 = call-poly <vilib>:"Mean.vi"("X"=w192) -> ("mean"=w189:dbl)  [unwired: 1 out]
                  n111 = case shown="\"Film Stable\"" "Humidity Status" {
                    selector: "Humidity Status" -> [w221 _ w228 _]
                    tunnel: w197 -> [w215 w227 w233 _]
                    tunnel: w195 -> [w216 _ _ _]
                    tunnel: "Hi Humidity Threshold (%)" -> [w223 _ _ _]
                    tunnel: "Low Humidity Threshold (%)" -> [w222 _ _ _]
                    tunnel: w189 -> [w217 _ _ _]
                    frame "Waiting For Film to Stabilize", Default {
                      n112 = Greater?(x=w216, y=w215) -> (0:w220:bool)
                      n113 = Less Or Equal?(x=w217, y=w223) -> (x <= y?=w210:bool)
                      n114 = Greater Or Equal?(x=w217, y=w222) -> (x >= y?=w212:bool)
                      n115 = Not And(1:w212, 2:w210) -> (0:w218:bool)
                      n116 = Select(t=u32 12386208, s=w210, f=u32 16711680) -> (s? t:f=w211:u32)
                      n117 = Select(t=u32 12386208, s=w212, f=u32 16711680) -> (s? t:f=w213:u32)
                      n118 = property on="Hi Humidity Threshold (%)" class="DigNum (strict)"("NumText.BG Color"=w211) -> ()  [unwired: 2 in, 2 out]
                      n119 = property on="Low Humidity Threshold (%)" class="DigNum (strict)"("NumText.BG Color"=w213) -> ()  [unwired: 2 in, 2 out]
                      n120 = And(x=w220, y=w218) -> (x .and. y?=w219:bool)
                      n121 = Select(t=w221, s=w219, f=T10."Exiting" ("Humidity Status")) -> (s? t:f=w224:u16)
                      n122 = local write "Humidity Status"(w224) -> ()
                    }
                    frame "Film Stable" {
                      n123 = Greater Or Equal?(x=w227, y=16) -> (x >= y?=w225:bool)
                      n124 = local write "Stable"(w225) -> ()
                    }
                    frame "Initializing" {
                      n125 = Less?(x=w233, y=16) -> (x < y?=w231:bool)
                      n126 = Select(t=w228, s=w231, f=T11."Waiting For Film to Stabilize" ("Humidity Status")) -> (s? t:f=w230:u16)
                      n127 = local write "Humidity Status"(w230) -> ()
                    }
                    frame "Exiting" {
                      n128 = property on="Stablizing" class="WFChart (strict)"("History Data"=dbl[][] []) -> ()  [unwired: 2 in, 2 out]
                      n129 = property on="Stable" class="Bool (strict)"("Visible"=TRUE) -> ()  [unwired: 2 in, 2 out]
                      n130 = local write "Humidity Status"(T6."Film Stable" ("Humidity Status")) -> ()
                    }
                  }
                }
              }
              n131 = local read "stage1 - humidity check"() -> (w157:i16[][])
              n132 = local read "Index"() -> (w156:u16)
            }
            frame "Calculating Target Voltages" {
              w237 = u8 0 ("Count")
              n133 = case shown="1" w242 {
                selector: w242 -> [w249 w281 w320]
                tunnel: w244 -> [w250 w264 w318]
                tunnel: [w250 w264 w317] -> w243
                tunnel: [w248 w278 w312] -> w241
                frame 0 {
                  n134 = property on="Stablizing" class="WFChart (strict)"() -> ("History Data"=w253:dbl[][])  [unwired: 2 in, 2 out]
                  n135 = local read "Cal Fail"() -> (w245:bool)
                  n136 = Index Array(array=w253, index (row)=4) -> (element=w256:dbl[])  [unwired: 1 in]
                  n137 = Index Array(array=w253, index (row)=5) -> (element=w255:dbl[])  [unwired: 1 in]
                  n138 = local read "Coefficients_In"() -> (w247:T2[])
                  n139 = property on="Cal Fail" class="Bool (strict)"("Visible"=w245, "Blinking"=w245) -> ()  [unwired: 2 in, 2 out]
                  n140 = call-poly <vilib>:"Mean.vi"("X"=w256) -> ("mean"=w252:dbl)  [unwired: 1 out]
                  n141 = call-poly <vilib>:"Mean.vi"("X"=w255) -> ("mean"=w251:dbl)  [unwired: 1 out]
                  n142 = for {
                    tunnel: w252 -> [w261]
                    tunnel: [w260] -> w246 mode=indexing
                    tunnel: w251 -> [w259]
                    tunnel: w247 -> [w258] mode=indexing
                    n143 = local write "Tcal_Chamber"(w261) -> ()
                    n144 = Bundle By Name(cluster=w258, "Chamber Temp"=w261, "Humidity"=w259) -> (w260:T2)
                    n145 = local write "Tcal_Humidity"(w259) -> ()
                  }
                  n146 = Increment(x=w249) -> (x+1=w248:u8)
                  n147 = local write "Coefficients_Out"(w246) -> ()
                }
                frame 1 {
                  n148 = local read "Coefficients_In"() -> (w280:T2[])
                  n149 = for {
                    tunnel: w280 -> [w307] mode=indexing
                    tunnel: [w306] -> w279 mode=indexing
                    tunnel: [w283] -> w277 mode=indexing
                    tunnel: [w290] -> w266 mode=indexing
                    tunnel: [w305] -> w276 mode=indexing
                    tunnel: [w304] -> w275 mode=indexing
                    tunnel: [w303] -> w274 mode=indexing
                    tunnel: [w298] -> w273 mode=indexing
                    tunnel: [w302] -> w269 mode=indexing
                    tunnel: [w301] -> w270 mode=indexing
                    tunnel: [w300] -> w271 mode=indexing
                    tunnel: [w299] -> w272 mode=indexing
                    tunnel: [w297] -> w268 mode=indexing
                    tunnel: [w291] -> w267 mode=indexing
                    tunnel: [w289] -> w265 mode=indexing
                    tunnel: [w284] -> w263 mode=indexing
                    tunnel: [w282] -> w262 mode=indexing
                    n150 = local read "Tcal_Chamber"() -> (w309:dbl)
                    n151 = local read "Calgas"() -> (w308:dbl)
                    n152 = call "Calculate C2V.vi"("Tcal_Chamber"=w309, "CO2"=w308, "Calibration Coefficients"=w307) -> ("Calibration Coefficients Out"=w292:T2)  [unwired: 8 in]
                    n153 = Unbundle By Name(w292) -> ("A"=w298:dbl, "B"=w303:dbl, "C"=w304:dbl, "D"=w305:dbl, "V6d"=w290:dbl, "V0d"=w289:dbl, "C2V"=w287:u16, "V2C"=w288:u16)
                    n154 = call "Calculate V2C.vi"("Tcal_Chamber"=w309, "Voltage In"=w290, "Calibration Coefficients"=w292) -> ("C'"=w294:dbl, "B'"=w295:dbl, "A'"=w296:dbl, "CO2 Out"=w291:dbl, "D'"=w293:dbl)  [unwired: 4 in]
                    n155 = call "Calculate V2C.vi"("Tcal_Chamber"=w309, "Voltage In"=w289, "Calibration Coefficients"=w292) -> ("C'"=w300:dbl, "B'"=w301:dbl, "A'"=w302:dbl, "CO2 Out"=w297:dbl, "D'"=w299:dbl)  [unwired: 4 in]
                    n156 = Subtract(x=w290, y=w289) -> (x-y=w283:dbl)
                    n157 = Equal To 0?(x=w287) -> (x = 0?=w285:bool)
                    n158 = Equal To 0?(x=w288) -> (x = 0?=w286:bool)
                    n159 = Not And(1:w286, 2:w285) -> (0:w284:bool)
                    n160 = Bundle By Name(cluster=w292, "C6d"=w291, "A'"=w296, "B'"=w295, "C'"=w294, "D'"=w293, "C0d"=w297) -> (w306:T2)
                    n161 = Less Than 0?(x=w283) -> (x < 0?=w282:bool)
                  }
                  "V_0d(target)" <- w265
                  "V_6d(target)" <- w266
                  "V_span(target)" <- w277
                  "C6FC2V" <- w267
                  "A" <- w273
                  "B" <- w274
                  "C" <- w275
                  "D" <- w276
                  "B'" <- w270
                  "C'" <- w271
                  "D'" <- w272
                  "A'" <- w269
                  "C0FC2V" <- w268
                  "Status" <- w263
                  "BlueLED" <- w262
                  "BlueLED 2" <- w262
                  "BlueLED 3" <- w262
                  n162 = Increment(x=w281) -> (x+1=w278:u8)
                  n163 = local write "Coefficients_Out"(w279) -> ()
                }
                frame 2, Default {
                  n164 = Increment(x=w318) -> (x+1=w316:T4)
                  n165 = Greater?(x=w320, y=u8 50) -> (0:w313:bool)
                  n166 = local read "Cal Fail"() -> (w310:bool)
                  n167 = Select(t=w316, s=w313, f=w318) -> (s? t:f=w317:T4)
                  n168 = Not(x=w313) -> (.not. x?=w311:bool)
                  n169 = Increment(x=w320) -> (x+1=w315:u8)
                  n170 = property on="Cal Fail" class="Bool (strict)"("Visible"=w310, "Blinking"=w310) -> ()  [unwired: 2 in, 2 out]
                  n171 = Select(t=w315, s=w311, f=u8 0) -> (s? t:f=w312:u8)
                }
              }
            }
            frame "Setting Zero Point" {
              w330 = 4 ("index")
              # "ZERO COMPLETE - MOVE TO NEXT SEQUENCE"
              n172 = Build Array(w334) -> (→"Zero":dbl[][])
              n173 = Initialize Array(0.015, w330) -> (w329:dbl[])
              n174 = Initialize Array(0.005, w330) -> (w328:dbl[])
              n175 = local read "Status"() -> (w325:bool[])
              n176 = local read "I_span"() -> (w326:dbl[])
              n177 = case shown="10" w324 {
                selector: w324 -> [_ w362 w373 w378 w399 w428 w434 w445 w450 w466 w503 w523 w533 w557 w562 _]
                tunnel: [1 w361 w371 w376 w398 w427 w433 w443 w448 w465 w504 w522 w532 w556 w561 0] -> w338
                tunnel: w344 -> [w353 w360 w370 w377 w400 w426 w432 w442 w449 w473 w506 w524 w531 w558 w563 w568]
                tunnel: [w353 w360 w370 w377 w400 w426 w432 w442 w449 w473 w506 w524 w531 w558 w563 w567] -> w343
                tunnel: 20 ("y") -> [_ _ w367 _ _ _ _ w439 _ _ _ _ _ _ _ _]
                tunnel: w337 -> [_ _ _ w375 w394 w422 w430 w436 w447 w472 w505 w525 w535 w552 w564 w566]
                tunnel: w336 -> [w349 w358 w366 _ _ _ _ _ _ _ _ _ _ _ _ _]
                tunnel: 5 ("index") -> [_ _ _ _ _ _ _ _ _ _ _ _ _ _ _ _]
                tunnel: u8 0 ("CalGasTank") -> [w351 _ _ _ _ w424 _ _ _ _ _ _ _ _ _ _]
                tunnel: w328 -> [w346 w354 w363 w374 w388 _ _ _ _ _ w501 _ _ _ _ _]
                tunnel: w329 -> [_ _ _ _ _ w421 w429 w435 w446 w460 w502 _ _ _ _ _]
                tunnel: [w349 w358 w366 w375 w394 w422 w430 w436 w447 w472 w505 w525 w535 w552 w564 w566] -> w335
                tunnel: w334 -> [_ _ _ _ w392 _ _ _ _ w464 _ _ _ _ _ _]
                tunnel: [w346 w354 w363 w374 w388 w421 w429 w435 w446 w460 w494 w520 w530 w559 w560 w565] -> w327
                tunnel: w326 -> [_ _ _ _ _ _ _ _ _ _ w494 w520 w530 w559 w560 w565]
                tunnel: w325 -> [_ _ _ _ w379 _ _ _ _ w451 w493 _ _ _ _ _]
                frame 0 {
                  w345 = FALSE ("Visible")
                  # "SET DAC AND GAS TANK"
                  n178 = local write "CalGasTank"(w351) -> ()
                  n179 = local write "SetDac"(TRUE ("InCal")) -> ()
                  n180 = property on="mI" class="Arr (strict)"("Visible"=w345) -> ()  [unwired: 2 in, 2 out]
                  n181 = property on="DAC scale" class="Arr (strict)"("Visible"=w345) -> ()  [unwired: 2 in, 2 out]
                  n182 = property on="BlueLED" class="Arr (strict)"("Visible"=w345) -> ()  [unwired: 2 in, 2 out]
                  n183 = property on="V_RA(5mA)" class="Arr (strict)"("Visible"=w345) -> ()  [unwired: 2 in, 2 out]
                  n184 = property on="V_RA(15mA)" class="Arr (strict)"("Visible"=w345) -> ()  [unwired: 2 in, 2 out]
                  n185 = property on="CHANNEL 2" class="Arr (strict)"("Visible"=w345) -> ()  [unwired: 2 in, 2 out]
                  n186 = Not(x=w345) -> (.not. x?=w347:bool)
                  n187 = property on="Zero" class="WFChart (strict)"("Visible"=w347) -> ()  [unwired: 2 in, 2 out]
                  "Zero Status" <- T7."Setting Zero at 5 mA" ("Zero Status")
                }
                frame 1 {
                  # "CLEAR HISTORY WRITE DAC"
                  n188 = Initialize Array(0, 4 ("dimension size")) -> (w356:i32[])
                  n189 = property on="Zero" class="WFChart (strict)"("History Data"=dbl[][] []) -> ()  [unwired: 2 in, 2 out]
                  n190 = local write "mI"(w356) -> ()
                  n191 = local write "V_RA(15mA)"(w356) -> ()
                  n192 = local write "V_RA(5mA)"(w356) -> ()
                  n193 = Increment(x=w362) -> (x+1=w361:u8)
                }
                frame 2 {
                  # "WAIT FOR FIRST1 SECS"
                  n194 = property on="Zero" class="WFChart (strict)"() -> ("History Data"=w368:dbl[][])  [unwired: 2 in, 2 out]
                  n195 = Array Size(array=w368) -> (size(s)=w365:i32[])
                  n196 = Add Array Elements(numeric array=w365) -> (sum=w364:i32)
                  n197 = Greater?(x=w364, y=w367) -> (0:w369:bool)
                  n198 = Increment(x=w373) -> (x+1=w372:u8)
                  n199 = Select(t=w372, s=w369, f=w373) -> (s? t:f=w371:u8)
                }
                frame 3 {
                  # "IGNORE FIRST1 SECS - RESET AIRFLOW"
                  n200 = Increment(x=w378) -> (x+1=w376:u8)
                }
                frame 4 {
                  # "RUN TEST UNTIL STABLE"
                  n201 = property on="Zero" class="WFChart (strict)"() -> ("History Data"=w390:dbl[][])  [unwired: 2 in, 2 out]
                  n202 = Transpose 2D Array(2D array=w390) -> (transposed array=w389:dbl[][])
                  n203 = for {
                    tunnel: w389 -> [w407] mode=indexing
                    tunnel: w392 -> [w406] mode=indexing
                    tunnel: [w405] -> w387 mode=indexing
                    tunnel: [w404] -> w391 mode=indexing
                    tunnel: [w403] -> w380 mode=indexing
                    tunnel: w379 -> [w402] mode=indexing
                    n204 = case shown="True" w402 {
                      tunnel: w407 -> [_ w415]
                      tunnel: w406 -> [_ w414]
                      tunnel: [TRUE w413] -> w405
                      tunnel: [0.0 ("mean") w412] -> w404
                      tunnel: [0.0 w411] -> w403
                      frame False {
                      }
                      frame True {
                        n205 = Reverse 1D Array(array=w415) -> (reversed array=w416:dbl[])
                        n206 = Split 1D Array(array=w416, index=16) -> (first subarray=w417:dbl[])  [unwired: 1 out]
                        n207 = call-poly <vilib>:"Mean.vi"("X"=w417) -> ("mean"=w412:dbl)  [unwired: 1 out]
                        n208 = Subtract(x=w412, y=w414) -> (x-y=w419:dbl)
                        n209 = Absolute Value(x=w419) -> (abs(x)=w411:dbl)
                        n210 = Less Or Equal?(x=w411, y=0.001) -> (x <= y?=w413:bool)
                      }
                    }
                  }
                  "V_RA(5mA)" <- w391
                  n211 = Array Size(array=w389) -> (size(s)=w397:i32[])
                  n212 = Add Array Elements(numeric array=w397) -> (sum=w382:i32)
                  n213 = Greater?(x=w382, y=40 ("index")) -> (0:w395:bool)
                  n214 = Increment(x=w399) -> (x+1=w401:u8)
                  n215 = Greater?(x=w382, y=100 ("index")) -> (0:w383:bool)
                  n216 = Add Array Elements(numeric array=w380) -> (sum=w381:dbl)
                  n217 = And Array Elements(Boolean array=w387) -> (logical AND=w386:bool)
                  n218 = local write "delta 2"(w381) -> ()
                  n219 = And(x=w395, y=w386) -> (x .and. y?=w384:bool)
                  n220 = Compound Arithmetic op=OR(w383, w384) -> (w393:bool)
                  n221 = Select(t=w401, s=w393, f=w399) -> (s? t:f=w398:u8)
                }
                frame 5 {
                  # "SET DAC AND GAS TANK"
                  n222 = local write "CalGasTank"(w424) -> ()
                  n223 = local write "SetDac"(TRUE ("InCal")) -> ()
                  n224 = local write "Zero Status"(T7."Setting Zero at 15 mA" ("Zero Status")) -> ()
                  n225 = Increment(x=w428) -> (x+1=w427:u8)
                }
                frame 6 {
                  # "CLEAR HISTORY WRITE DAC"
                  n226 = property on="Zero" class="WFChart (strict)"("History Data"=dbl[][] []) -> ()  [unwired: 2 in, 2 out]
                  n227 = Increment(x=w434) -> (x+1=w433:u8)
                }
                frame 7 {
                  # "WAIT FOR FIRST 1 SECS"
                  n228 = property on="Zero" class="WFChart (strict)"() -> ("History Data"=w440:dbl[][])  [unwired: 2 in, 2 out]
                  n229 = Array Size(array=w440) -> (size(s)=w441:i32[])
                  n230 = Add Array Elements(numeric array=w441) -> (sum=w438:i32)
                  n231 = Greater?(x=w438, y=w439) -> (0:w437:bool)
                  n232 = Increment(x=w445) -> (x+1=w444:u8)
                  n233 = Select(t=w444, s=w437, f=w445) -> (s? t:f=w443:u8)
                }
                frame 8 {
                  # "IGNORE FIRST 1 SECS - RESET AIRFLOW"
                  n234 = Increment(x=w450) -> (x+1=w448:u8)
                }
                frame 9 {
                  # "RUN TEST UNTIL STABLE"
                  n235 = property on="Zero" class="WFChart (strict)"() -> ("History Data"=w462:dbl[][])  [unwired: 2 in, 2 out]
                  n236 = Transpose 2D Array(2D array=w462) -> (transposed array=w461:dbl[][])
                  n237 = for {
                    tunnel: w461 -> [w479] mode=indexing
                    tunnel: w464 -> [w478] mode=indexing
                    tunnel: [w477] -> w459 mode=indexing
                    tunnel: [w476] -> w463 mode=indexing
                    tunnel: [w475] -> w452 mode=indexing
                    tunnel: w451 -> [w474] mode=indexing
                    n238 = case shown="True" w474 {
                      tunnel: w479 -> [_ w487]
                      tunnel: w478 -> [_ w486]
                      tunnel: [TRUE w485] -> w477
                      tunnel: [0.0 ("mean") w484] -> w476
                      tunnel: [0.0 w483] -> w475
                      frame False {
                      }
                      frame True {
                        n239 = Reverse 1D Array(array=w487) -> (reversed array=w488:dbl[])
                        n240 = Split 1D Array(array=w488, index=16) -> (first subarray=w489:dbl[])  [unwired: 1 out]
                        n241 = call-poly <vilib>:"Mean.vi"("X"=w489) -> ("mean"=w484:dbl)  [unwired: 1 out]
                        n242 = Subtract(x=w484, y=w486) -> (x-y=w491:dbl)
                        n243 = Absolute Value(x=w491) -> (abs(x)=w483:dbl)
                        n244 = Less Or Equal?(x=w483, y=0.001) -> (x <= y?=w485:bool)
                      }
                    }
                  }
                  "V_RA(15mA)" <- w463
                  n245 = Array Size(array=w461) -> (size(s)=w470:i32[])
                  n246 = Add Array Elements(numeric array=w470) -> (sum=w455:i32)
                  n247 = Greater?(x=w455, y=40 ("index")) -> (0:w468:bool)
                  n248 = Increment(x=w466) -> (x+1=w471:u8)
                  n249 = Greater?(x=w455, y=100 ("index")) -> (0:w454:bool)
                  n250 = Add Array Elements(numeric array=w452) -> (sum=→"delta 2":dbl)
                  n251 = And Array Elements(Boolean array=w459) -> (logical AND=w458:bool)
                  n252 = And(x=w468, y=w458) -> (x .and. y?=w457:bool)
                  n253 = Compound Arithmetic op=OR(w454, w457) -> (w467:bool)
                  n254 = Select(t=w471, s=w467, f=w466) -> (s? t:f=w465:u8)
                }
                frame 10 {
                  # "CALCULATE"
                  n255 = Subtract(x=w502, y=w501) -> (x-y=w500:dbl[])
                  n256 = local read "V_RA(15mA)"() -> (w498:dbl[])
                  n257 = local read "V_RA(5mA)"() -> (w499:dbl[])
                  n258 = for {
                    tunnel: w500 -> [w510] mode=indexing
                    tunnel: w499 -> [w511] mode=indexing
                    tunnel: w498 -> [w512] mode=indexing
                    tunnel: [w509] -> w497 mode=indexing
                    tunnel: [0.0 ("x*y")] -> w495 mode=indexing
                    tunnel: w493 -> [w507] mode=indexing
                    n259 = case shown="True" w507 {
                      tunnel: w512 -> [_ w518]
                      tunnel: w511 -> [_ w517]
                      tunnel: w510 -> [_ w515]
                      tunnel: [0.0 w514] -> w509
                      frame False {
                      }
                      frame True {
                        n260 = Subtract(x=w518, y=w517) -> (x-y=w516:dbl)
                        n261 = Divide(x=w516, y=w515) -> (x/y=w514:dbl)
                      }
                    }
                  }
                  "mI" <- w497
                  "I_delta" <- w495
                  n262 = local write "Zero Status"(T7."Calculating slopes" ("Zero Status")) -> ()
                  n263 = Increment(x=w503) -> (x+1=w504:u8)
                }
                frame 11 {
                  w519 = TRUE ("Visible")
                  # "ZERO COMPLETE - Display and wait one sec"
                  n264 = property on="mI" class="Arr (strict)"("Visible"=w519) -> ()  [unwired: 2 in, 2 out]
                  n265 = property on="BlueLED" class="Arr (strict)"("Visible"=w519) -> ()  [unwired: 2 in, 2 out]
                  n266 = property on="DAC scale" class="Arr (strict)"("Visible"=w519) -> ()  [unwired: 2 in, 2 out]
                  n267 = property on="V_RA(5mA)" class="Arr (strict)"("Visible"=w519) -> ()  [unwired: 2 in, 2 out]
                  n268 = property on="V_RA(15mA)" class="Arr (strict)"("Visible"=w519) -> ()  [unwired: 2 in, 2 out]
                  n269 = property on="CHANNEL 2" class="Arr (strict)"("Visible"=w519) -> ()  [unwired: 2 in, 2 out]
                  n270 = Not(x=w519) -> (.not. x?=w521:bool)
                  n271 = property on="Zero" class="WFChart (strict)"("Visible"=w521) -> ()  [unwired: 2 in, 2 out]
                  n272 = Increment(x=w523) -> (x+1=w522:u8)
                }
                frame 12 {
                  n273 = local write "OK 9"(FALSE) -> ()
                  n274 = local read "Coefficients_In"() -> (w539:T2[])
                  n275 = local read "V_RA(15mA)"() -> (w536:dbl[])
                  n276 = local read "V_RA(5mA)"() -> (w537:dbl[])
                  n277 = local read "BlueLED"() -> (w526:bool[])
                  n278 = local read "mI"() -> (w540:dbl[])
                  n279 = for {
                    tunnel: w540 -> [w544] mode=indexing
                    tunnel: w539 -> [w551] mode=indexing
                    tunnel: [w550] -> w538 mode=indexing
                    tunnel: w537 -> [w549] mode=indexing
                    tunnel: w536 -> [w548] mode=indexing
                    tunnel: [0.0] -> w529 mode=indexing
                    tunnel: [i8 0 ("Step")] -> w534 mode=indexing
                    tunnel: [w543] -> w528 mode=indexing
                    tunnel: [w542] -> w527 mode=indexing
                    tunnel: w526 -> [w542] mode=indexing
                    n280 = Bundle By Name(cluster=w551, "V_(RA,5mA)"=w549, "V_(RA,15mA)"=w548, "mI"=w544) -> (w550:T2)
                    n281 = Divide(x=50, y=w544) -> (x/y=w543:dbl)
                  }
                  "DAC scale" <- w528
                  "I'mBlue" <- w527
                  n282 = Increment(x=w533) -> (x+1=w532:u8)
                  n283 = local write "Step"(w534) -> ()
                  n284 = local write "I_delta"(w529) -> ()
                  n285 = local write "Coefficients_Out"(w538) -> ()
                }
                frame 13 {
                  # "Set DAC to start calgas early"
                  n286 = local read "I_span"() -> (w554:dbl[])
                  n287 = local write "SetDac"(TRUE ("InCal")) -> ()
                  n288 = local write "DAC Currents"(w554) -> ()
                  n289 = local read "Gas Tank"() -> (w555:u8)
                  n290 = local write "CalGasTank"(w555) -> ()
                  n291 = Increment(x=w557) -> (x+1=w556:u8)
                }
                frame 14, Default {
                  # "ZERO COMPLETE - Display and wait one sec"
                  n292 = Increment(x=w562) -> (x+1=w561:u8)
                }
                frame 30 {
                  n293 = Increment(x=w568) -> (x+1=w567:T4)
                }
              }
              n294 = local write "DAC Currents"(w327) -> ()
              n295 = local read "stage 2 - zeroing"() -> (w323:i16[][])
              n296 = local read "Index"() -> (w321:u16)
            }
            frame "Setting High Point" {
              w581 = 4 ("index")
              # "ZERO COMPLETE - MOVE TO NEXT SEQUENCE"
              n297 = Build Array(w584) -> (→"Zero 3":dbl[][])
              n298 = Initialize Array(0.005, w581) -> (w579:dbl[])
              n299 = Initialize Array(0.015, w581) -> (w580:dbl[])
              n300 = local read "Status"() -> (w576:bool[])
              n301 = local read "I_span"() -> (w577:dbl[])
              n302 = case shown="13" w575 {
                selector: w575 -> [_ w605 w623 w634 w639 w660 w689 w695 w706 w711 w727 w764 w784 w794 w818 w823 _]
                tunnel: [1 w606 w622 w632 w637 w659 w688 w694 w704 w709 w726 w765 w783 w793 w817 w822 0] -> w588
                tunnel: w593 -> [w603 w604 w621 w631 w638 w661 w687 w693 w703 w710 w734 w767 w785 w792 w819 w824 w829]
                tunnel: [w603 w604 w621 w631 w638 w661 w687 w693 w703 w710 w734 w767 w785 w792 w819 w824 w828] -> w592
                tunnel: 20 ("y") -> [_ _ _ w628 _ _ _ _ w700 _ _ _ _ _ _ _ _]
                tunnel: w587 -> [_ _ _ _ w636 w655 w683 w691 w697 w708 w733 w766 w786 w796 w813 w825 w827]
                tunnel: w586 -> [w599 w613 w619 w627 _ _ _ _ _ _ _ _ _ _ _ _ _]
                tunnel: 5 ("index") -> [_ _ _ _ _ _ _ _ _ _ _ _ _ _ _ _ _]
                tunnel: "Gas Tank" -> [w601 _ _ _ _ _ w685 _ _ _ _ _ _ _ _ _ _]
                tunnel: w579 -> [w596 _ w615 w624 w635 w649 _ _ _ _ _ w762 _ _ _ _ _]
                tunnel: w580 -> [_ _ _ _ _ _ w682 w690 w696 w707 w721 w763 _ _ _ _ _]
                tunnel: [w599 w613 w619 w627 w636 w655 w683 w691 w697 w708 w733 w766 w786 w796 w813 w825 w827] -> w585
                tunnel: w584 -> [_ _ _ _ _ w653 _ _ _ _ w725 _ _ _ _ _ _]
                tunnel: [w596 w614 w615 w624 w635 w649 w682 w690 w696 w707 w721 w755 w781 w791 w820 w821 w826] -> w578
                tunnel: w577 -> [_ w614 _ _ _ _ _ _ _ _ _ w755 w781 w791 w820 w821 w826]
                tunnel: w576 -> [_ _ _ _ _ w640 _ _ _ _ w712 w754 _ _ _ _ _]
                frame 0 {
                  w595 = FALSE ("Visible")
                  # "SET DAC AND GAS TANK"
                  # "SET DAC AND GAS TANK"
                  n303 = local write "CalGasTank"(w601) -> ()
                  n304 = local write "SetDac"(TRUE ("InCal")) -> ()
                  n305 = property on="mI 2" class="Arr (strict)"("Visible"=w595) -> ()  [unwired: 2 in, 2 out]
                  n306 = property on="BlueLED" class="Arr (strict)"("Visible"=w595) -> ()  [unwired: 2 in, 2 out]
                  n307 = property on="Zero 3" class="WFChart (strict)"("History Data"=dbl[][] []) -> ()  [unwired: 2 in, 2 out]
                  n308 = property on="V_RA(5mA) 2" class="Arr (strict)"("Visible"=w595) -> ()  [unwired: 2 in, 2 out]
                  n309 = property on="V_RA(15mA) 2" class="Arr (strict)"("Visible"=w595) -> ()  [unwired: 2 in, 2 out]
                  n310 = property on="DAC scale 2" class="Arr (strict)"("Visible"=w595) -> ()  [unwired: 2 in, 2 out]
                  n311 = property on="CHANNEL 3" class="Arr (strict)"("Visible"=w595) -> ()  [unwired: 2 in, 2 out]
                  n312 = Not(x=w595) -> (.not. x?=w597:bool)
                  n313 = property on="Zero 3" class="WFChart (strict)"("Visible"=w597) -> ()  [unwired: 2 in, 2 out]
                  "Zero Status 2" <- T8."Setting High at 5 mA" ("Zero Status 2")
                }
                frame 1 {
                  n314 = property on="Zero 3" class="WFChart (strict)"() -> ("History Data"=w612:dbl[][])  [unwired: 2 in, 2 out]
                  n315 = Array Size(array=w612) -> (size(s)=w611:i32[])
                  n316 = Increment(x=w605) -> (x+1=w609:u8)
                  n317 = Add Array Elements(numeric array=w611) -> (sum=w607:i32)
                  n318 = Greater?(x=w607, y=10) -> (0:w608:bool)
                  n319 = Select(t=w609, s=w608, f=w605) -> (s? t:f=w606:u8)
                }
                frame 2 {
                  # "CLEAR HISTORY WRITE DAC"
                  n320 = Initialize Array(0, 4 ("dimension size")) -> (w617:i32[])
                  n321 = property on="Zero 3" class="WFChart (strict)"("History Data"=dbl[][] []) -> ()  [unwired: 2 in, 2 out]
                  n322 = local write "mI 2"(w617) -> ()
                  n323 = local write "V_RA(15mA) 2"(w617) -> ()
                  n324 = local write "V_RA(5mA) 2"(w617) -> ()
                  n325 = Increment(x=w623) -> (x+1=w622:u8)
                }
                frame 3 {
                  # "WAIT FOR FIRST1 SECS"
                  n326 = property on="Zero 3" class="WFChart (strict)"() -> ("History Data"=w629:dbl[][])  [unwired: 2 in, 2 out]
                  n327 = Array Size(array=w629) -> (size(s)=w626:i32[])
                  n328 = Add Array Elements(numeric array=w626) -> (sum=w625:i32)
                  n329 = Greater?(x=w625, y=w628) -> (0:w630:bool)
                  n330 = Increment(x=w634) -> (x+1=w633:u8)
                  n331 = Select(t=w633, s=w630, f=w634) -> (s? t:f=w632:u8)
                }
                frame 4 {
                  # "IGNORE FIRST1 SECS - RESET AIRFLOW"
                  n332 = Increment(x=w639) -> (x+1=w637:u8)
                }
                frame 5 {
                  # "RUN TEST UNTIL STABLE"
                  n333 = property on="Zero 3" class="WFChart (strict)"() -> ("History Data"=w651:dbl[][])  [unwired: 2 in, 2 out]
                  n334 = Transpose 2D Array(2D array=w651) -> (transposed array=w650:dbl[][])
                  n335 = for {
                    tunnel: w650 -> [w668] mode=indexing
                    tunnel: w653 -> [w667] mode=indexing
                    tunnel: [w666] -> w648 mode=indexing
                    tunnel: [w665] -> w652 mode=indexing
                    tunnel: [w664] -> w641 mode=indexing
                    tunnel: w640 -> [w663] mode=indexing
                    n336 = case shown="True" w663 {
                      tunnel: w668 -> [_ w676]
                      tunnel: w667 -> [_ w675]
                      tunnel: [TRUE w674] -> w666
                      tunnel: [0.0 ("mean") w673] -> w665
                      tunnel: [0.0 w672] -> w664
                      frame False {
                      }
                      frame True {
                        n337 = Reverse 1D Array(array=w676) -> (reversed array=w677:dbl[])
                        n338 = Split 1D Array(array=w677, index=16) -> (first subarray=w678:dbl[])  [unwired: 1 out]
                        n339 = call-poly <vilib>:"Mean.vi"("X"=w678) -> ("mean"=w673:dbl)  [unwired: 1 out]
                        n340 = Subtract(x=w673, y=w675) -> (x-y=w680:dbl)
                        n341 = Absolute Value(x=w680) -> (abs(x)=w672:dbl)
                        n342 = Less Or Equal?(x=w672, y=0.001) -> (x <= y?=w674:bool)
                      }
                    }
                  }
                  "V_RA(5mA) 2" <- w652
                  n343 = Array Size(array=w650) -> (size(s)=w658:i32[])
                  n344 = Add Array Elements(numeric array=w658) -> (sum=w643:i32)
                  n345 = Greater?(x=w643, y=40 ("index")) -> (0:w656:bool)
                  n346 = Increment(x=w660) -> (x+1=w662:u8)
                  n347 = Greater?(x=w643, y=100 ("index")) -> (0:w644:bool)
                  n348 = Add Array Elements(numeric array=w641) -> (sum=w642:dbl)
                  n349 = And Array Elements(Boolean array=w648) -> (logical AND=w647:bool)
                  n350 = local write "delta 3"(w642) -> ()
                  n351 = And(x=w656, y=w647) -> (x .and. y?=w645:bool)
                  n352 = Compound Arithmetic op=OR(w644, w645) -> (w654:bool)
                  n353 = Select(t=w662, s=w654, f=w660) -> (s? t:f=w659:u8)
                }
                frame 6 {
                  # "SET DAC AND GAS TANK"
                  n354 = local write "CalGasTank"(w685) -> ()
                  n355 = local write "SetDac"(TRUE ("InCal")) -> ()
                  n356 = local write "Zero Status 2"(T8."Setting High at 15 mA" ("Zero Status 2")) -> ()
                  n357 = Increment(x=w689) -> (x+1=w688:u8)
                }
                frame 7 {
                  # "CLEAR HISTORY WRITE DAC"
                  n358 = property on="Zero 3" class="WFChart (strict)"("History Data"=dbl[][] []) -> ()  [unwired: 2 in, 2 out]
                  n359 = Increment(x=w695) -> (x+1=w694:u8)
                }
                frame 8 {
                  # "WAIT FOR FIRST 1 SECS"
                  n360 = property on="Zero 3" class="WFChart (strict)"() -> ("History Data"=w701:dbl[][])  [unwired: 2 in, 2 out]
                  n361 = Array Size(array=w701) -> (size(s)=w702:i32[])
                  n362 = Add Array Elements(numeric array=w702) -> (sum=w699:i32)
                  n363 = Greater?(x=w699, y=w700) -> (0:w698:bool)
                  n364 = Increment(x=w706) -> (x+1=w705:u8)
                  n365 = Select(t=w705, s=w698, f=w706) -> (s? t:f=w704:u8)
                }
                frame 9 {
                  # "IGNORE FIRST 1 SECS - RESET AIRFLOW"
                  n366 = Increment(x=w711) -> (x+1=w709:u8)
                }
                frame 10 {
                  # "RUN TEST UNTIL STABLE"
                  n367 = property on="Zero 3" class="WFChart (strict)"() -> ("History Data"=w723:dbl[][])  [unwired: 2 in, 2 out]
                  n368 = Transpose 2D Array(2D array=w723) -> (transposed array=w722:dbl[][])
                  n369 = for {
                    tunnel: w722 -> [w740] mode=indexing
                    tunnel: w725 -> [w739] mode=indexing
                    tunnel: [w738] -> w720 mode=indexing
                    tunnel: [w737] -> w724 mode=indexing
                    tunnel: [w736] -> w713 mode=indexing
                    tunnel: w712 -> [w735] mode=indexing
                    n370 = case shown="True" w735 {
                      tunnel: w740 -> [_ w748]
                      tunnel: w739 -> [_ w747]
                      tunnel: [TRUE w746] -> w738
                      tunnel: [0.0 ("mean") w745] -> w737
                      tunnel: [0.0 w744] -> w736
                      frame False {
                      }
                      frame True {
                        n371 = Reverse 1D Array(array=w748) -> (reversed array=w749:dbl[])
                        n372 = Split 1D Array(array=w749, index=16) -> (first subarray=w750:dbl[])  [unwired: 1 out]
                        n373 = call-poly <vilib>:"Mean.vi"("X"=w750) -> ("mean"=w745:dbl)  [unwired: 1 out]
                        n374 = Subtract(x=w745, y=w747) -> (x-y=w752:dbl)
                        n375 = Absolute Value(x=w752) -> (abs(x)=w744:dbl)
                        n376 = Less Or Equal?(x=w744, y=0.001) -> (x <= y?=w746:bool)
                      }
                    }
                  }
                  "V_RA(15mA) 2" <- w724
                  n377 = Array Size(array=w722) -> (size(s)=w731:i32[])
                  n378 = Add Array Elements(numeric array=w731) -> (sum=w716:i32)
                  n379 = Greater?(x=w716, y=40 ("index")) -> (0:w729:bool)
                  n380 = Increment(x=w727) -> (x+1=w732:u8)
                  n381 = Greater?(x=w716, y=100 ("index")) -> (0:w715:bool)
                  n382 = Add Array Elements(numeric array=w713) -> (sum=→"delta 3":dbl)
                  n383 = And Array Elements(Boolean array=w720) -> (logical AND=w719:bool)
                  n384 = And(x=w729, y=w719) -> (x .and. y?=w718:bool)
                  n385 = Compound Arithmetic op=OR(w715, w718) -> (w728:bool)
                  n386 = Select(t=w732, s=w728, f=w727) -> (s? t:f=w726:u8)
                }
                frame 11 {
                  # "CALCULATE"
                  n387 = Subtract(x=w763, y=w762) -> (x-y=w761:dbl[])
                  n388 = local read "V_RA(15mA) 2"() -> (w759:dbl[])
                  n389 = local read "V_RA(5mA) 2"() -> (w760:dbl[])
                  n390 = local write "Zero Status 2"(T8."Calculating slopes" ("Zero Status 2")) -> ()
                  n391 = for {
                    tunnel: w761 -> [w771] mode=indexing
                    tunnel: w760 -> [w772] mode=indexing
                    tunnel: w759 -> [w773] mode=indexing
                    tunnel: [w770] -> w758 mode=indexing
                    tunnel: [0.0 ("x*y")] -> w756 mode=indexing
                    tunnel: w754 -> [w768] mode=indexing
                    n392 = case shown="True" w768 {
                      tunnel: w773 -> [_ w779]
                      tunnel: w772 -> [_ w778]
                      tunnel: w771 -> [_ w776]
                      tunnel: [0.0 w775] -> w770
                      frame False {
                      }
                      frame True {
                        n393 = Subtract(x=w779, y=w778) -> (x-y=w777:dbl)
                        n394 = Divide(x=w777, y=w776) -> (x/y=w775:dbl)
                      }
                    }
                  }
                  "mI 2" <- w758
                  "I_delta 2" <- w756
                  n395 = Increment(x=w764) -> (x+1=w765:u8)
                }
                frame 12 {
                  w780 = TRUE ("Visible")
                  # "ZERO COMPLETE - Display and wait one sec"
                  n396 = property on="mI 2" class="Arr (strict)"("Visible"=w780) -> ()  [unwired: 2 in, 2 out]
                  n397 = property on="BlueLED" class="Arr (strict)"("Visible"=w780) -> ()  [unwired: 2 in, 2 out]
                  n398 = property on="V_RA(5mA) 2" class="Arr (strict)"("Visible"=w780) -> ()  [unwired: 2 in, 2 out]
                  n399 = property on="V_RA(15mA) 2" class="Arr (strict)"("Visible"=w780) -> ()  [unwired: 2 in, 2 out]
                  n400 = property on="DAC scale 2" class="Arr (strict)"("Visible"=w780) -> ()  [unwired: 2 in, 2 out]
                  n401 = property on="CHANNEL 3" class="Arr (strict)"("Visible"=w780) -> ()  [unwired: 2 in, 2 out]
                  n402 = Not(x=w780) -> (.not. x?=w782:bool)
                  n403 = property on="Zero 3" class="WFChart (strict)"("Visible"=w782) -> ()  [unwired: 2 in, 2 out]
                  n404 = Increment(x=w784) -> (x+1=w783:u8)
                }
                frame 13 {
                  n405 = local write "OK 9"(FALSE) -> ()
                  n406 = local read "Coefficients_In"() -> (w800:T2[])
                  n407 = local read "V_RA(15mA) 2"() -> (w797:dbl[])
                  n408 = local read "V_RA(5mA) 2"() -> (w798:dbl[])
                  n409 = local read "BlueLED"() -> (w787:bool[])
                  n410 = local read "mI 2"() -> (w801:dbl[])
                  n411 = for {
                    tunnel: w801 -> [w805] mode=indexing
                    tunnel: w800 -> [w812] mode=indexing
                    tunnel: [w811] -> w799 mode=indexing
                    tunnel: w798 -> [w810] mode=indexing
                    tunnel: w797 -> [w809] mode=indexing
                    tunnel: [0.0] -> w790 mode=indexing
                    tunnel: [i8 0 ("Step")] -> w795 mode=indexing
                    tunnel: [w804] -> w789 mode=indexing
                    tunnel: [w803] -> w788 mode=indexing
                    tunnel: w787 -> [w803] mode=indexing
                    n412 = Bundle By Name(cluster=w812, "V_(RA,5mA)"=w810, "V_(RA,15mA)"=w809, "mI"=w805) -> (w811:T2)
                    n413 = Divide(x=50, y=w805) -> (x/y=w804:dbl)
                  }
                  "DAC scale 2" <- w789
                  "I'mBlue 2" <- w788
                  n414 = Increment(x=w794) -> (x+1=w793:u8)
                  n415 = local write "Step"(w795) -> ()
                  n416 = local write "Coefficients_Out"(w799) -> ()
                  n417 = local write "I_delta 2"(w790) -> ()
                }
                frame 14 {
                  # "Set DAC to start calgas early"
                  n418 = local read "I_span"() -> (w815:dbl[])
                  n419 = local write "SetDac"(TRUE ("InCal")) -> ()
                  n420 = local write "DAC Currents"(w815) -> ()
                  n421 = local read "Gas Tank"() -> (w816:u8)
                  n422 = local write "CalGasTank"(w816) -> ()
                  n423 = Increment(x=w818) -> (x+1=w817:u8)
                }
                frame 15, Default {
                  # "ZERO COMPLETE - Display and wait one sec"
                  n424 = Increment(x=w823) -> (x+1=w822:u8)
                }
                frame 30 {
                  n425 = Increment(x=w829) -> (x+1=w828:T4)
                }
              }
              n426 = local write "DAC Currents"(w578) -> ()
              n427 = local read "stage 2 - zeroing"() -> (w574:i16[][])
              n428 = local read "Index"() -> (w572:u16)
            }
            frame "Setting Span Point" {
              n429 = Build Array(w844) -> (→"Span Point Calibration":dbl[][])
              n430 = local read "V_span(target)"() -> (w841:dbl[])
              n431 = local read "V_span(ImA)"() -> (w840:dbl[])
              n432 = local read "V_0d(ImA)"() -> (w843:dbl[])
              n433 = local read "DAC scale"() -> (w837:dbl[])
              n434 = local read "Gas Tank"() -> (w831:u8)
              n435 = local read "I'mBlue"() -> (w838:bool[])
              n436 = local read "Status"() -> (w839:bool[])
              n437 = Subtract(x=w841, y=w840) -> (x-y=w842:dbl[])
              n438 = local read "DAC"() -> (w836:u16[])
              n439 = case shown="0, Default" w835 {
                selector: w835 -> [w864 w881 w893 w895 w917 w956 w985 w996 w1050 w1082 w1124 w1128 w1132 w1136 w1140 _]
                tunnel: "OK 9" -> [_ _ _ _ _ w952 _ _ _ w1081 _ _ _ _ _ _]
                tunnel: [w863 w884 w892 w894 w918 w957 w984 w994 w1049 w1083 w1123 w1127 w1131 w1135 w1139 0 ("Step")] -> w849
                tunnel: w853 -> [w866 w888 w891 w903 w920 w960 w983 w995 w1048 w1087 w1121 w1125 w1129 w1133 w1137 w1143]
                tunnel: [w866 w888 w891 w903 w920 w960 w983 w995 w1048 w1087 w1121 w1125 w1129 w1133 w1137 w1141] -> w852
                tunnel: w847 -> [w865 w880 w889 _ _ _ _ _ _ _ _ _ _ _ _ _]
                tunnel: w848 -> [_ _ _ w902 w914 w950 w982 w986 w1047 w1072 w1122 w1126 w1130 w1134 w1138 w1144]
                tunnel: w841 -> [_ _ _ _ w904 _ _ w993 w1042 w1080 _ _ _ _ _ _]
                tunnel: w831 -> [w861 _ _ _ _ _ _ _ _ _ _ _ _ _ _ _]
                tunnel: [w865 w880 w889 w902 w914 w950 w982 w986 w1047 w1072 w1122 w1126 w1130 w1134 w1138 w1144] -> w846
                tunnel: w844 -> [_ _ _ _ w911 w949 _ _ _ _ _ _ _ _ _ _]
                tunnel: w843 -> [_ _ _ _ w910 w945 _ _ w1038 _ _ _ _ _ _ _]
                tunnel: w840 -> [_ _ _ _ _ _ _ w990 w1041 w1079 _ _ _ _ _ _]
                tunnel: w839 -> [w855 _ _ _ w905 w940 _ w989 w1040 w1070 _ _ _ _ _ _]
                tunnel: w838 -> [_ _ _ _ _ _ _ w988 _ _ _ _ _ _ _ _]
                tunnel: w837 -> [_ _ _ _ _ _ _ w987 _ _ _ _ _ _ _ _]
                tunnel: w836 -> [_ _ _ _ _ _ _ _ w1039 w1071 _ _ _ _ _ _]
                frame 0, Default {
                  # "SET DAC AND GAS TANK"
                  n440 = local write "CalGasTank"(w861) -> ()
                  n441 = local read "I_span"() -> (w859:dbl[])
                  n442 = local read "I_delta"() -> (w858:dbl[])
                  n443 = local read "mI"() -> (w860:dbl[])
                  n444 = local write "SetDac"(TRUE ("InCal")) -> ()
                  n445 = for {
                    tunnel: w860 -> [w870] mode=indexing
                    tunnel: [w869] -> w854 mode=indexing
                    tunnel: w859 -> [w872] mode=indexing
                    tunnel: w858 -> [w871] mode=indexing
                    tunnel: [w868] -> w857 mode=indexing
                    tunnel: [w868] -> w856 mode=indexing
                    tunnel: w855 -> [w867] mode=indexing
                    n446 = case shown="True" w867 {
                      tunnel: w872 -> [_ w878]
                      tunnel: w871 -> [_ w877]
                      tunnel: w870 -> [_ w876]
                      tunnel: [w873 w875] -> w869
                      tunnel: [w873 w874] -> w868
                      frame False {
                        w873 = 0.0
                      }
                      frame True {
                        n447 = Add(x=w878, y=w877) -> (x+y=w874:dbl)
                        n448 = Multiply(x=w874, y=w876) -> (x*y=w875:dbl)
                      }
                    }
                  }
                  "V_0d(ImA)" <- w854
                  n449 = Increment(x=w864) -> (x+1=w863:u8)
                  n450 = local write "I_span"(w856) -> ()
                  n451 = local write "DAC Currents"(w857) -> ()
                }
                frame 1 {
                  # "Wait half a sec"
                  n452 = Increment(x=w881) -> (x+1=w883:u8)
                  n453 = property on="Span Point Calibration" class="WFChart (strict)"() -> ("History Data"=w887:dbl[][])  [unwired: 2 in, 2 out]
                  n454 = Array Size(array=w887) -> (size(s)=w886:i32[])
                  n455 = Add Array Elements(numeric array=w886) -> (sum=w879:i32)
                  n456 = Greater?(x=w879, y=10) -> (0:w882:bool)
                  n457 = Select(t=w883, s=w882, f=w881) -> (s? t:f=w884:u8)
                }
                frame 2 {
                  # "CLEAR HISTORY WRITE DAC"
                  # "Discard dac settling data"
                  n458 = property on="Span Point Calibration" class="WFChart (strict)"("History Data"=dbl[][] []) -> ()  [unwired: 2 in, 2 out]
                  n459 = Increment(x=w893) -> (x+1=w892:u8)
                }
                frame 3 {
                  # "Now accumulate one sec of data into buffer for mean calculation"
                  n460 = property on="Span Point Calibration" class="WFChart (strict)"() -> ("History Data"=w901:dbl[][])  [unwired: 2 in, 2 out]
                  n461 = Array Size(array=w901) -> (size(s)=w900:i32[])
                  n462 = Add Array Elements(numeric array=w900) -> (sum=w896:i32)
                  n463 = Increment(x=w895) -> (x+1=w898:u8)
                  n464 = Greater?(x=w896, y=20) -> (0:w897:bool)
                  n465 = Select(t=w898, s=w897, f=w895) -> (s? t:f=w894:u8)
                }
                frame 4 {
                  # "QUICK CHECK"
                  # "QUICK CHECK - that mean is within 1V of target - if any are not readjust and re-loop"
                  n466 = property on="Span Point Calibration" class="WFChart (strict)"() -> ("History Data"=w907:dbl[][])  [unwired: 2 in, 2 out]
                  n467 = Transpose 2D Array(2D array=w907) -> (transposed array=w906:dbl[][])
                  n468 = for {
                    tunnel: w906 -> [w926] mode=indexing
                    tunnel: [w928] -> w909 mode=indexing
                    tunnel: w911 -> [w927] mode=indexing
                    tunnel: [w924] -> w912 mode=indexing
                    tunnel: [w925] -> w913 mode=indexing
                    tunnel: w910 -> [w923] mode=indexing
                    tunnel: w905 -> [w922] mode=indexing
                    tunnel: w904 -> [w921] mode=indexing
                    n469 = case shown="True" w922 {
                      tunnel: [FALSE w939] -> w928
                      tunnel: w927 -> [_ _]
                      tunnel: w926 -> [_ w938]
                      tunnel: [w930 w937] -> w925
                      tunnel: [w930 w931] -> w924
                      tunnel: w923 -> [_ w936]
                      tunnel: w921 -> [_ w932]
                      frame False {
                        w930 = 0.0
                      }
                      frame True {
                        n470 = call-poly <vilib>:"Mean.vi"("X"=w938) -> ("mean"=w937:dbl)  [unwired: 1 out]
                        n471 = Subtract(x=w937, y=w936) -> (x-y=w931:dbl)
                        n472 = Subtract(x=w931, y=w932) -> (x-y=w933:dbl)
                        n473 = Absolute Value(x=w933) -> (abs(x)=w934:dbl)
                        n474 = Less Or Equal?(x=w934, y=1.0) -> (x <= y?=w939:bool)
                      }
                    }
                  }
                  n475 = Increment(x=w917) -> (x+1=w919:u8)
                  n476 = Add(x=w917, y=2) -> (x+y=w915:i32)
                  n477 = local write "V_6d(ImA)"(w913) -> ()
                  n478 = local write "V_span(ImA)"(w912) -> ()
                  n479 = Or Array Elements(Boolean array=w909) -> (logical OR=w908:bool)
                  n480 = Select(t=w919, s=w908, f=w915) -> (s? t:f=w918:i32)
                }
                frame 5 {
                  # "RUN TEST UNTIL STABLE"
                  # "We are within a volt for all channels so now check for stable signals"
                  n481 = property on="Span Point Calibration" class="WFChart (strict)"() -> ("History Data"=w944:dbl[][])  [unwired: 2 in, 2 out]
                  n482 = Transpose 2D Array(2D array=w944) -> (transposed array=w943:dbl[][])
                  n483 = for {
                    tunnel: w943 -> [w967] mode=indexing
                    tunnel: [w966] -> w942 mode=indexing
                    tunnel: w949 -> [w965] mode=indexing
                    tunnel: [w964] -> w948 mode=indexing
                    tunnel: [w963] -> w946 mode=indexing
                    tunnel: w945 -> [w962] mode=indexing
                    tunnel: w940 -> [w961] mode=indexing
                    n484 = case shown="True" w961 {
                      tunnel: w967 -> [_ w975]
                      tunnel: [FALSE w974] -> w966
                      tunnel: w965 -> [_ w973]
                      tunnel: [w969 w972] -> w964
                      tunnel: [w969 w970] -> w963
                      tunnel: w962 -> [_ w971]
                      frame False {
                        w969 = 0.0 ("mean")
                      }
                      frame True {
                        n485 = Reverse 1D Array(array=w975) -> (reversed array=w976:dbl[])
                        n486 = Split 1D Array(array=w976, index=16) -> (first subarray=w977:dbl[])  [unwired: 1 out]
                        n487 = call-poly <vilib>:"Mean.vi"("X"=w977) -> ("mean"=w970:dbl)  [unwired: 1 out]
                        n488 = Subtract(x=w970, y=w973) -> (x-y=w979:dbl)
                        n489 = Subtract(x=w970, y=w971) -> (x-y=w972:dbl)
                        n490 = Absolute Value(x=w979) -> (abs(x)=w980:dbl)
                        n491 = Less Or Equal?(x=w980, y=0.005) -> (x <= y?=w974:bool)
                      }
                    }
                  }
                  "V_span(ImA)" <- w948
                  "V_6d(ImA)" <- w946
                  n492 = Array Size(array=w943) -> (size(s)=w954:i32[])
                  n493 = Add Array Elements(numeric array=w954) -> (sum=w947:i32)
                  n494 = Greater?(x=w947, y=100 ("index")) -> (0:w953:bool)
                  n495 = Or(x=w952, y=w953) -> (x .or. y?=w951:bool)
                  n496 = Increment(x=w956) -> (x+1=w959:u8)
                  n497 = Or Array Elements(Boolean array=w942) -> (logical OR=w941:bool)
                  n498 = Or(x=w951, y=w941) -> (x .or. y?=w958:bool)
                  n499 = Select(t=w959, s=w958, f=w956) -> (s? t:f=w957:u8)
                }
                frame 6 {
                  n500 = Increment(x=w985) -> (x+1=w984:u8)
                }
                frame 7 {
                  # "CALCULATE"
                  n501 = for {
                    tunnel: w993 -> [w1001] mode=indexing
                    tunnel: [w1003] -> w992 mode=indexing
                    tunnel: [w1002] -> w991 mode=indexing
                    tunnel: w990 -> [w1000] mode=indexing
                    tunnel: w989 -> [w999] mode=indexing
                    tunnel: w988 -> [w998] mode=indexing
                    tunnel: w987 -> [w997] mode=indexing
                    n502 = case shown="True" w999 {
                      tunnel: [0.0 w1025] -> w1003
                      tunnel: [i8 0 ("t") w1006] -> w1002
                      tunnel: w1001 -> [_ w1024]
                      tunnel: w1000 -> [_ w1023]
                      tunnel: w998 -> [_ w1019]
                      tunnel: w997 -> [_ w1018]
                      frame False {
                      }
                      frame True {
                        # "Scale DAC"
                        n503 = Subtract(x=w1024, y=w1023) -> (x-y=w1030:dbl)
                        n504 = Less Than 0?(x=w1030) -> (x < 0?=w1016:bool)
                        n505 = Absolute Value(x=w1030) -> (abs(x)=w1011:dbl)
                        n506 = Not(x=w1016) -> (.not. x?=w1015:bool)
                        n507 = Less Or Equal?(x=w1011, y=0.1) -> (x <= y?=w1036:bool)
                        n508 = Less Or Equal?(x=w1011, y=0.25) -> (x <= y?=w1031:bool)
                        n509 = Select(t=w1015, s=w1019, f=w1016) -> (s? t:f=w1021:bool)
                        n510 = Select(t=i8 1, s=w1036, f=i8 3 ("t")) -> (s? t:f=w1020:i8)
                        n511 = Select(t=w1020, s=w1031, f=i8 10 ("t")) -> (s? t:f=w1027:i8)
                        n512 = Less Or Equal?(x=w1011, y=1.0) -> (x <= y?=w1012:bool)
                        n513 = Less Or Equal?(x=w1011, y=0.5) -> (x <= y?=w1010:bool)
                        n514 = Select(t=w1027, s=w1010, f=i8 30 ("t")) -> (s? t:f=w1009:i8)
                        n515 = Select(t=w1009, s=w1012, f=i8 60 ("t")) -> (s? t:f=w1008:i8)
                        n516 = Multiply(x=w1018, y=w1008) -> (x*y=w1017:dbl)
                        n517 = Negate(x=w1017) -> (-x=w1022:dbl)
                        n518 = Select(t=w1022, s=w1021, f=w1017) -> (s? t:f=w1007:dbl)
                        n519 = To Word Integer(number=w1007) -> (16bit integer=w1006:i16)
                        n520 = Multiply(x=0.0001 ("y"), y=w1006) -> (x*y=w1025:dbl)
                      }
                    }
                  }
                  "Step" <- w991
                  n521 = Increment(x=w996) -> (x+1=w994:u8)
                  n522 = local write "I_delta"(w992) -> ()
                }
                frame 8 {
                  # "Coarse update to approx CO2 calc"
                  n523 = local read "Coefficients_In"() -> (w1046:T2[])
                  n524 = local read "V_0d(target)"() -> (w1043:dbl[])
                  n525 = local read "I_span"() -> (w1044:dbl[])
                  n526 = for {
                    tunnel: w1046 -> [w1060] mode=indexing
                    tunnel: [w1059] -> w1045 mode=indexing
                    tunnel: w1039 -> [w1058] mode=indexing
                    tunnel: w1044 -> [w1057] mode=indexing
                    tunnel: w1038 -> [w1056] mode=indexing
                    tunnel: w1043 -> [w1052] mode=indexing
                    tunnel: w1042 -> [w1055] mode=indexing
                    tunnel: w1041 -> [w1053] mode=indexing
                    tunnel: w1040 -> [w1054] mode=indexing
                    n527 = case shown="True" w1054 {
                      tunnel: [w1063 w1069] -> w1062
                      tunnel: [w1063 w1068] -> w1061
                      tunnel: w1056 -> [_ w1067]
                      tunnel: w1052 -> [_ w1066]
                      tunnel: w1055 -> [_ w1065]
                      tunnel: w1053 -> [_ w1064]
                      frame False {
                        w1063 = 0.0
                      }
                      frame True {
                        n528 = Subtract(x=w1067, y=w1066) -> (x-y=w1068:dbl)
                        n529 = Divide(x=w1065, y=w1064) -> (x/y=w1069:dbl)
                      }
                    }
                    n530 = Add(x=w1052, y=w1053) -> (x+y=w1051:dbl)
                    n531 = Bundle By Name(cluster=w1060, "V_6d_ImA (actual)"=w1051, "DAC"=w1058, "I_span"=w1057, "V_offs"=w1061, "G_adj"=w1062) -> (w1059:T2)
                  }
                  n532 = Increment(x=w1050) -> (x+1=w1049:u8)
                  n533 = local write "Coefficients_Out"(w1045) -> ()
                }
                frame 9 {
                  # "CALCULATE"
                  n534 = local read "I_delta"() -> (w1075:dbl[])
                  n535 = local read "Step"() -> (w1078:i16[])
                  n536 = for {
                    tunnel: w1080 -> [w1102] mode=indexing
                    tunnel: w1079 -> [w1101] mode=indexing
                    tunnel: w1078 -> [w1100] mode=indexing
                    tunnel: [w1096] -> w1073 mode=indexing
                    tunnel: [w1099] -> w1076 mode=indexing
                    tunnel: w1075 -> [w1098] mode=indexing
                    tunnel: [w1097] -> w1074 mode=indexing
                    tunnel: w1071 -> [w1092] mode=indexing
                    tunnel: [w1089] -> _ mode=indexing
                    tunnel: w1070 -> [w1089] mode=indexing
                    n537 = Equal?(x=w1092, y=u16 1023) -> (x = y?=w1094:bool)
                    n538 = Equal To 0?(x=w1092) -> (x = 0?=w1095:bool)
                    n539 = Or(x=w1095, y=w1094) -> (x .or. y?=w1091:bool)
                    n540 = Not(x=w1091) -> (.not. x?=w1090:bool)
                    n541 = And(x=w1090, y=w1089) -> (x .and. y?=w1088:bool)
                    n542 = case shown="True" w1088 {
                      tunnel: w1102 -> [_ w1113]
                      tunnel: w1101 -> [_ w1112]
                      tunnel: w1100 -> [_ w1111]
                      tunnel: [i8 0 ("Step") w1110] -> w1099
                      tunnel: w1098 -> [_ w1109]
                      tunnel: [0.0 ("V_(RA,5mA)") w1107] -> w1097
                      tunnel: [TRUE w1106] -> w1096
                      frame False {
                      }
                      frame True {
                        w1108 = i8 0 ("t")
                        n543 = Subtract(x=w1113, y=w1112) -> (x-y=w1114:dbl)
                        n544 = Absolute Value(x=w1114) -> (abs(x)=w1115:dbl)
                        n545 = Less?(x=w1115, y=0.05) -> (x < y?=w1106:bool)
                        n546 = Select(t=w1108, s=w1106, f=w1111) -> (s? t:f=w1110:i16)
                        n547 = Select(t=w1108, s=w1106, f=w1109) -> (s? t:f=w1107:dbl)
                      }
                    }
                  }
                  n548 = Increment(x=w1082) -> (x+1=w1085:u8)
                  n549 = local write "Step"(w1076) -> ()
                  n550 = local write "I_delta"(w1074) -> ()
                  n551 = local write "Span Good"(w1073) -> ()
                  n552 = And Array Elements(Boolean array=w1073) -> (logical AND=w1077:bool)
                  n553 = Or(x=w1081, y=w1077) -> (x .or. y?=w1084:bool)
                  n554 = Select(t=w1085, s=w1084, f=0) -> (s? t:f=w1083:i32)
                }
                frame 10 {
                  # "Just delay a few counts to allow storage of a few correct CO2s"
                  n555 = local write "CalGasTank"(u8 0 ("CalGasTank")) -> ()
                  n556 = local write "SetDac"(TRUE ("InCal")) -> ()
                  n557 = local write "OK 10"(FALSE ("OK 10")) -> ()
                  n558 = property on="Zero Offset" class="WFChart (strict)"("History Data"=dbl[][] []) -> ()  [unwired: 2 in, 2 out]
                  n559 = Increment(x=w1124) -> (x+1=w1123:u8)
                }
                frame 11 {
                  # "Just delay a few counts to allow storage of a few correct CO2s"
                  n560 = Increment(x=w1128) -> (x+1=w1127:u8)
                }
                frame 12 {
                  # "Just delay a few counts to allow storage of a few correct CO2s"
                  n561 = Increment(x=w1132) -> (x+1=w1131:u8)
                }
                frame 13 {
                  # "Just delay a few counts to allow storage of a few correct CO2s"
                  n562 = Increment(x=w1136) -> (x+1=w1135:u8)
                }
                frame 14 {
                  # "Just delay a few counts to allow storage of a few correct CO2s"
                  n563 = Increment(x=w1140) -> (x+1=w1139:u8)
                }
                frame 15 {
                  # "Now Exit"
                  n564 = Increment(x=w1143) -> (x+1=w1141:T4)
                }
              }
              n565 = local write "V_Span Delta"(w842) -> ()
              n566 = local read "stage 3 - span"() -> (w834:i16[][])
              n567 = local read "Index"() -> (w833:u16)
            }
            frame "Calculating Gain & Offset" {
              w1155 = u16 450  # Fast AirPump
              n568 = property on="DAC Currents" class="Arr (strict)"("Visible"=TRUE) -> ()  [unwired: 2 in, 2 out]
              n569 = Build Array(w1151) -> (→"Zero Offset":dbl[][])
              n570 = local read "Status"() -> (w1149:bool[])
              n571 = case shown="0, Default" w1147 {
                selector: w1147 -> [_ w1167 w1177 w1181 w1191 w1221 _]
                tunnel: [1 w1166 w1175 w1179 w1190 w1225 1] -> w1157
                tunnel: w1159 -> [w1163 w1165 w1174 w1180 w1192 w1226 w1248]
                tunnel: [w1163 w1165 w1174 w1180 w1192 w1226 w1247] -> w1158
                tunnel: w1154 -> [_ _ _ w1178 w1183 _ _]
                tunnel: w1155 -> [w1161 w1164 w1169 _ _ _ _]
                tunnel: [w1161 w1164 w1169 w1178 w1183 w1217 w1245] -> w1156
                tunnel: w1153 -> [_ _ _ _ _ w1217 w1245]
                tunnel: w1151 -> [_ _ _ _ w1186 _ _]
                tunnel: w1149 -> [_ _ _ _ w1182 w1209 _]
                frame 0, Default {
                  # "SET DAC AND GAS TANK\n\nMOVED TO END OF SPAN TO SHOW FINAL NUMBERS"
                }
                frame 1 {
                  # "CLEAR HISTORY WRITE DAC"
                  n572 = Increment(x=w1167) -> (x+1=w1166:u8)
                }
                frame 2 {
                  # "WAIT FOR FIRST 5 SECS"
                  n573 = property on="Zero Offset" class="WFChart (strict)"() -> ("History Data"=w1171:dbl[][])  [unwired: 2 in, 2 out]
                  n574 = Array Size(array=w1171) -> (size(s)=w1173:i32[])
                  n575 = Add Array Elements(numeric array=w1173) -> (sum=w1168:i32)
                  n576 = Increment(x=w1177) -> (x+1=w1176:u8)
                  n577 = Greater?(x=w1168, y=40) -> (0:w1172:bool)
                  n578 = Select(t=w1176, s=w1172, f=w1177) -> (s? t:f=w1175:u8)
                }
                frame 3 {
                  # "IGNORE FIRST 2 SECS - RESET AIRFLOW"
                  n579 = Increment(x=w1181) -> (x+1=w1179:u8)
                }
                frame 4 {
                  # "RUN TEST UNTIL STABLE"
                  n580 = property on="Zero Offset" class="WFChart (strict)"() -> ("History Data"=w1189:dbl[][])  [unwired: 2 in, 2 out]
                  n581 = Transpose 2D Array(2D array=w1189) -> (transposed array=w1188:dbl[][])
                  n582 = for {
                    tunnel: w1188 -> [w1197] mode=indexing
                    tunnel: [w1196] -> w1187 mode=indexing
                    tunnel: w1186 -> [w1195] mode=indexing
                    tunnel: [w1194] -> w1185 mode=indexing
                    tunnel: w1182 -> [w1193] mode=indexing
                    n583 = case shown="False" w1193 {
                      tunnel: w1197 -> [_ w1202]
                      tunnel: [w1198 w1201] -> w1196
                      tunnel: w1195 -> [_ w1200]
                      tunnel: [w1198 w1199] -> w1194
                      frame False {
                        w1198 = 0.0 ("mean")
                      }
                      frame True {
                        n584 = Reverse 1D Array(array=w1202) -> (reversed array=w1203:dbl[])
                        n585 = Split 1D Array(array=w1203, index=16) -> (first subarray=w1204:dbl[])  [unwired: 1 out]
                        n586 = call-poly <vilib>:"Mean.vi"("X"=w1204) -> ("mean"=w1201:dbl)  [unwired: 1 out]
                        n587 = Subtract(x=w1201, y=w1200) -> (x-y=w1206:dbl)
                        n588 = Absolute Value(x=w1206) -> (abs(x)=w1199:dbl)
                      }
                    }
                  }
                  n589 = Increment(x=w1191) -> (x+1=w1190:u8)
                  n590 = Add Array Elements(numeric array=w1185) -> (sum=→"delta":dbl)
                  n591 = local write "V_0d(ImA)"(w1187) -> ()
                }
                frame 5 {
                  # "CALCULATE"
                  n592 = local read "V_span(target)"() -> (w1211:dbl[])
                  n593 = local read "V_0d(target)"() -> (w1212:dbl[])
                  n594 = local read "V_6d(ImA)"() -> (w1210:dbl[])
                  n595 = local read "V_0d(ImA)"() -> (w1213:dbl[])
                  n596 = for {
                    tunnel: [w1235] -> w1216 mode=indexing
                    tunnel: [w1234] -> w1215 mode=indexing
                    tunnel: [w1233] -> w1214 mode=indexing
                    tunnel: w1213 -> [w1232] mode=indexing
                    tunnel: w1211 -> [w1231] mode=indexing
                    tunnel: w1212 -> [w1230] mode=indexing
                    tunnel: w1210 -> [w1229] mode=indexing
                    tunnel: [w1228] -> w1208 mode=indexing
                    tunnel: w1209 -> [w1227] mode=indexing
                    n597 = case shown="True" w1227 {
                      tunnel: [w1236 w1244] -> w1235
                      tunnel: [w1236 w1243] -> w1234
                      tunnel: [w1236 w1242] -> w1233
                      tunnel: w1232 -> [_ w1241]
                      tunnel: w1231 -> [_ w1240]
                      tunnel: w1230 -> [_ w1239]
                      tunnel: w1229 -> [_ w1238]
                      tunnel: [w1236 0.001] -> w1228
                      frame False {
                        w1236 = 0.0
                      }
                      frame True {
                        n598 = Subtract(x=w1241, y=w1239) -> (x-y=w1242:dbl)
                        n599 = Subtract(x=w1238, y=w1241) -> (x-y=w1243:dbl)
                        n600 = Divide(x=w1240, y=w1243) -> (x/y=w1244:dbl)
                      }
                    }
                  }
                  "V_0(adjust)" <- w1214
                  "V_span(adjust)" <- w1215
                  "Gain(adjust)" <- w1216
                  n601 = Increment(x=w1221) -> (x+1=w1223:u8)
                  n602 = Decrement(x=w1221) -> (x-1=w1222:u8)
                  n603 = Add Array Elements(numeric array=w1208) -> (sum=w1207:dbl)
                  n604 = local read "delta"() -> (w1224:dbl)
                  n605 = Less Or Equal?(x=w1224, y=w1207) -> (x <= y?=w1220:bool)
                  n606 = Or(x=w1220, y="OK 10") -> (x .or. y?=w1219:bool)
                  n607 = Select(t=w1223, s=w1219, f=w1222) -> (s? t:f=w1225:u8)
                }
                frame 6 {
                  # "GAIN & OFFSET COMPLETE - MOVE TO NEXT SEQUENCE"
                  n608 = call <vilib>:"Beep.vi"() -> ()  [unwired: 12 in]
                  n609 = Increment(x=w1248) -> (x+1=w1247:T4)
                }
              }
              n610 = local read "stage 4 - offset adjust"() -> (w1148:i16[][])
              n611 = local read "Index"() -> (w1146:u16)
            }
            frame "Storing Calibration Coefficients" {
              w1249 = 0
              n612 = case shown="1" w1254 {
                selector: w1254 -> [w1267 w1292 w1325 w1331]
                tunnel: w1259 -> [w1271 w1290 w1323 w1336]
                tunnel: [w1266 w1290 w1323 w1335] -> w1258
                tunnel: w1257 -> [w1273 w1298 w1327 w1334]
                tunnel: [w1270 w1297 w1326 w1333] -> w1256
                tunnel: w1255 -> [w1272 w1286 w1322 w1329]
                tunnel: [w1267 w1291 w1324 w1330] -> w1253
                tunnel: [w1272 w1286 w1322 w1329] -> w1252
                tunnel: w1251 -> [w1268 w1287 _ _]
                frame 0 {
                  w1265 = FALSE ("Visible")
                  # "This case is only reached when skip calibration is selected at the start"
                  n613 = local write "Quit"(TRUE ("Cal Fail")) -> ()
                  n614 = local read "time_now"() -> (w1269:timestamp)
                  n615 = property on="Quit" class="Bool (strict)"("Visible"=w1265) -> ()  [unwired: 2 in, 2 out]
                  n616 = local read "Coefficients_In"() -> (w1262:T2[])
                  n617 = Subtract(x=w1269, y=w1268) -> (x-y=w1264:dbl)
                  n618 = property on="elapsed time" class="DigNum (strict)"("Visible"=w1265) -> ()  [unwired: 2 in, 2 out]
                  n619 = for {
                    tunnel: w1264 -> [w1276]
                    tunnel: "CAL SKIPPED" -> [w1277]
                    tunnel: w1262 -> [w1275] mode=indexing
                    tunnel: [w1274] -> w1261 mode=indexing
                    n620 = Bundle By Name(cluster=w1275, "cal_utc"=w1276, "zero_utc"=w1276, "TYPE"=w1277) -> (w1274:T2)
                  }
                  n621 = Decrement(x=w1273) -> (x-1=w1270:u16)
                  n622 = Increment(x=w1271) -> (x+1=w1266:T4)
                  n623 = local write "Coefficients_Out"(w1261) -> ()
                }
                frame 1 {
                  w1283 = TRUE ("want seconds? (F)")
                  n624 = local read "time_now"() -> (w1289:timestamp)
                  "Calibration Complete -" <- w1289
                  n625 = Subtract(x=w1289, y=w1287) -> (x-y=w1288:dbl)
                  n626 = local read "Coefficients_In"() -> (w1284:T2[])
                  n627 = local read "elapsed time"() -> (w1293:i16)
                  "duration" <- w1293
                  n628 = local read "Gain(adjust)"() -> (w1280:dbl[])
                  n629 = local read "V_0(adjust)"() -> (w1281:dbl[])
                  n630 = local read "V_0d(ImA)"() -> (w1282:dbl[])
                  n631 = local read "V_6d(ImA)"() -> (w1279:dbl[])
                  n632 = Get Date/Time String(date format (0)=enum16{"short", "long", "abbreviated"}."short", seconds (now)=w1289, want seconds? (F)=w1283) -> (date string=w1294:string, time string=w1295:string)
                  n633 = local read "Status"() -> (w1278:bool[])
                  n634 = for {
                    tunnel: w1283 -> [_]
                    tunnel: w1295 -> [w1303]
                    tunnel: w1294 -> [w1305]
                    tunnel: w1293 -> [w1301]
                    tunnel: w1288 -> [w1307]
                    tunnel: w1286 -> [w1314]
                    tunnel: [w1313] -> w1285 mode=indexing
                    tunnel: w1284 -> [w1312] mode=indexing
                    tunnel: w1282 -> [w1299] mode=indexing
                    tunnel: w1281 -> [w1311] mode=indexing
                    tunnel: w1280 -> [w1310] mode=indexing
                    tunnel: w1279 -> [w1309] mode=indexing
                    tunnel: w1278 -> [w1308] mode=indexing
                    n635 = case shown="False" w1308 {
                      tunnel: [0.0 w1321] -> w1306
                      tunnel: w1307 -> [_ w1321]
                      tunnel: w1305 -> [_ w1320]
                      tunnel: [w1315 w1320] -> w1304
                      tunnel: w1303 -> [_ w1319]
                      tunnel: [w1315 w1319] -> w1302
                      tunnel: w1301 -> [_ w1318]
                      tunnel: [i16 0 ("elapsed time") w1318] -> w1300
                      frame False {
                        w1315 = ""
                      }
                      frame True {
                      }
                    }
                    n636 = Bundle By Name(cluster=w1312, "cal_utc"=w1306, "CalDate"=w1304, "CalTime"=w1302, "duration"=w1300, "V_(()d, average)"=w1299, "V_0d_ImA (actual)"=w1299, "V_6d_ImA (actual)"=w1309, "cal_offs_adj"=w1311, "cal_gain_adj"=w1310, "V_offs"=w1311, "G_adj"=w1310, "Pump Flow Rate"=w1314) -> (w1313:T2)
                  }
                  n637 = Decrement(x=w1298) -> (x-1=w1297:u16)
                  n638 = Increment(x=w1292) -> (x+1=w1291:u8)
                  n639 = local write "Coefficients_Out"(w1285) -> ()
                }
                frame 2, Default {
                  n640 = Decrement(x=w1327) -> (x-1=w1326:u16)
                  n641 = Increment(x=w1325) -> (x+1=w1324:u8)
                }
                frame 20 {
                  w1332 = FALSE ("Visible")
                  n642 = property class="VI"("Exec.CloseFPAfterCall"=TRUE ("Execution:Close After Call")) -> ()  [unwired: 2 in, 2 out]
                  n643 = property on="Quit" class="Bool (strict)"("Visible"=w1332) -> ()  [unwired: 2 in, 2 out]
                  n644 = property on="elapsed time" class="DigNum (strict)"("Visible"=w1332) -> ()  [unwired: 2 in, 2 out]
                  n645 = Decrement(x=w1334) -> (x-1=w1333:u16)
                  n646 = Increment(x=w1336) -> (x+1=w1335:T4)
                  n647 = Increment(x=w1331) -> (x+1=w1330:u8)
                }
              }
            }
            frame "Calibration Complete" {
              w1337 = 0 ("Count")
              w1339 = TRUE
              n648 = property class="VI"("Exec.CloseFPAfterCall"=w1339) -> ()  [unwired: 2 in, 2 out]
              n649 = case shown="True" w1339 {
                frame False {
                }
                frame True {
                  n650 = local write "Quit"(FALSE) -> ()
                  n651 = property class="VI"("FP.State"=T9."Closed" ("Front Panel Window:State")) -> ()  [unwired: 2 in, 2 out]
                }
              }
              n652 = Decrement(x=w1343) -> (x-1=w1342:u16)
              "Calibration Complete" <- w1339
            }
          }
          "Count" <- w48
          "Actual" <- w46
          n653 = call "Get Pump Sequence.vi"("Array"=w38, "Index"=w40, "Stage"=w41) -> ("Error"=→"Error":bool, "Pump Settings"=→"Pump Settings":T1, "Updated Index"=→"Index":u16, "Ignore"=w35:bool)  [unwired: 5 in]
          n654 = Not(x=w35) -> (.not. x?=w34:bool)
          n655 = property on="Pump Settings" class="Clust (strict)"("Visible"=w34) -> ()  [unwired: 2 in, 2 out]
        }
        frame True {
          w1347 = FALSE ("Calibration Complete")
          n656 = property class="VI"("Exec.CloseFPAfterCall"=w1347, "FP.State"=T9."Standard" ("Front Panel Window:State")) -> ()  [unwired: 2 in, 2 out]
          n657 = property on="Pump Settings" class="Clust (strict)"("Visible"=w1347) -> ()  [unwired: 2 in, 2 out]
        }
      }
      "Progress Out" <- w33
      "CalStatus Out" <- w31
      n658 = Not(x="SetDac In Process") -> (.not. x?=w21:bool)
      n659 = property on="Span Point Calibration" class="WFChart (strict)"("Visible"=w21) -> ()  [unwired: 2 in, 2 out]
      n660 = local write "Progress"(w33) -> ()
    }
    frame #2 {
    }
  }
